vi "Text control 2 v2.9.vi"() -> ()   [LabVIEW 2016]
panel:
  in  "Start Time":dbl caption="Set Start Time (s)"
  out "Total lines":i32
  out "Line running":i32
  in  "byte count":u32=64
  in  "Serial Settings:Serial End Mode for Reads":u16(ring)=2 items=["None", "LastBit", "TermChar"]
  in  "Timeout (ms)":u32=10000
  in  "Enable Termination\nChar (T)":bool=TRUE
  in  "Termination char\n(0xA = '\\n' = LF)\n(0xD = '\\r' = CR)":u8=13 format="%.0x"
  in  "flow control":u16(ring) items=["None"=0, "XON/XOFF"=1, "RTS/CTS"=2, "DTR/DSR"=4]
  in  "stop bits":u16(ring)=10 items=["1.0"=10, "1.5"=15, "2.0"=20]
  in  "parity":u16(ring) items=["None", "Odd", "Even", "Mark", "Space"]
  in  "data bits":u16=8 min=5 max=8 step=1
  in  "VISA resource name":refnum<visa-resource-name>="COM6"
  in  "baud rate":u32=9600
  out "Serial port output":string
  out "error out":errorcluster
  in  "Units":u16(ring) items=["Seconds", "Minutes", "Hours"]
  out "Elapsed Time":dbl caption="Elapsed Time (s)"
  out "Id max vs time":cluster{"Y data in":dbl[], "X data in":dbl[]}[](graph)
  out "Ig":dbl format="%.2e"
  out "Id":dbl format="%.2e"
  out "Is":dbl format="%.2e"
  out "I vs Vg":cluster{"Y data in":dbl[], "X data in":dbl[]}[](graph)
  in  "Panel Controls 2":T1={"Emergency Stop"=refnum, "TransGraph Max"=1e-05, "Text/Graph (text=false)"=TRUE, "TransGraph Min"=1e-11} {"TransGraph Min" format="%.2e"; "TransGraph Max" format="%.2e"}
  out "Command running:":string="#output s 0 0 0 -0.008 0.008 0.002"
  in  "Standby":T2
  in  "Full Reset":bool
  in  "SMU4":cluster{"on/off":bool, "Voltage":dbl} {"Voltage" min=-100.0 max=100.0 format="%.2f"}
  in  "Source/Drain Range":u8(slide)=6 max=11 scale=0.0..11.0
  in  "Source/Drain\nRange mode":u16(ring) items=["Auto", "Limited", "Fixed"]
  in  "Gate Range":u8(slide)=6 max=11 scale=0.0..11.0
  in  "Gate Range\nmode":u16(ring) items=["Auto", "Limited", "Fixed"]
  in  "Gate":T3={"Gate Start"=0.0, "Gate Stop"=2.0, "Gate Step (linear only)"=1.0, "Gate Compliance"=0.0001, "Gate PComp"=0.0, "Range mode"=0, "Range"=6} {"Range" max=11 scale=0.0..11.0; "Range mode" items=["Auto", "Limited", "Fixed"]; "Gate PComp" format="%^.2e"; "Gate Compliance" format="%^.2e"; "Gate Step (linear only)" format="%^.4e"; "Gate Stop" format="%^.4e"; "Gate Start" format="%^.4e"}
  in  "Drain 2":T4={"Drain Start"=0.0, "Drain Stop"=2.0, "Drain Compliance"=0.0001, "Drain Step"=1.0, "Drain PComp"=0.0, "Range mode"=0, "Range"=6} {"Range" max=11 scale=0.0..11.0; "Range mode" items=["Auto", "Limited", "Fixed"]; "Drain PComp" format="%^.2e"; "Drain Step" format="%^.4e"; "Drain Compliance" format="%^.2e"; "Drain Stop" format="%^.4e"; "Drain Start" format="%^.4e"}
  in  "Timings 2":T5={"integration time"=0, "Short/Long integration time"=0.00064, "hold time (sec)"=0.0, "delay time (sec)"=0.0, "Step Time (0 disables)"=0.0, "sweep method"=0, "Pulse period"=0.005, "Base voltage"=0.0, "Pulse width"=0.0005} {"Pulse width" min=0.0005 max=0.1 step=0.0001 format="%.4f"; "Base voltage" format="%^.4e"; "Pulse period" min=0.005 max=1.0 step=0.0001 format="%.4f"; "sweep method" items=["Continuous", "Pulsed"]; "Step Time (0 disables)" format="%.2f"; "delay time (sec)" format="%.4f"; "hold time (sec)" format="%.4f"; "Short/Long integration time" format="%^.0e"; "integration time" scale=0.0..2.0}
  in  "Panel Controls":T6={"Emergency Stop"=refnum, "TransGraph Max"=1e-05, "Text/Graph (text=false)"=TRUE} {"TransGraph Max" format="%.2e"}
  in  "Interrupt run":bool
  in  "Drain: Compliance":dbl=0.001 format="%.8f"
  in  "Gate: Compliance":dbl=0.001 format="%.8f"
  out "Path":path=path "C:/users/rlp38/09Apr2009LTtesting/test2.txt"
  in  "hold time /s":dbl format="%.2f"
  in  "delay time /s":dbl format="%.2f"
  in  "integration time":u32(slide) max=2 step=1 scale=0.0..2.0
  in  "Integration time (short)":dbl=0.0019 min=8e-05 max=0.0019 step=8e-05 format="%^.0e"
  in  "Integration time (long)":dbl=0.32 min=0.04 max=2.0 step=0.02 format="%.2f"
  in  "Step delay /s":dbl format="%.2f"
  in  "Program":string="#pulsedstressV d 0.03 20 0 0.5 0.0827 5\n#\n#itime s\n#gaterangemode l\n#drainrangemode l\n#pulsed on 0.05 0 0.02\n#transfer d 1 -1 -0.1 -1 -1 0\n#wait-min 1\n#transfer d 1 -1 -0.1 -1 -1 0\n#output d 0 -1 -0.5 0 -1 -0.1\n#transfer d -10 40 1 5 40 35\n#transfer d -10 40 1 5 40 35\n#output d 0 40 20 0 40 1\n#\n#\n#sample 1 0.008 221 6 0.003\n#samplei 400e-6 200 6 0.002 0.1\n#vsu2pulse -10 4\n#\n#stressV 0.016 0.03 2e-4 0.1e-3 11\n#stressI 220e-7 0.08 15\n#transfer s -1 1 0.5 -0.005 0.005 0.005\n#output s 0 0 0 -0.008 0.008 0.002\n"
  # "Serial port settings"
  # "Time"
  # "100 samples is approx 13s with medium integration"
  # "Syntax:\nitime [s|m|l]\ngaterangemode [a|l|f]\ndrainrangemode [a|l|f]\npulsed [on|off] PulsePeriod(sec) PulseBaseVoltage PulseONWidth(sec)\nstandby [on l off]\nwait NumMilliseconds\nwait-min NumMinutes\n# texthere = comment\ntransfer [s|d] VgStart VgStop VgStep VdStart VdStop VdStep\noutput [s|d] VgStart VgStop VgStep VdStart VdStop VdStep\nsample Vg Vd NumSamples Time(s) SampleInterval(s)\nsamplei Idg NumSamples Time(s) SampleInterval(s) VDGcompliance\n# if in doubt use SampleInterval(s) = 0.004\nstressV VG VD IGcompliance IDcompliance Duration(sec)\nstressI IDG VDGcompliance Duration(sec)\nvsu2pulse Bias Duration(s)\npulsedstressV [s|d] VEstop VgON VgOFF Period(s) PulseONwidth(s) Vd\nsample-fpp Vg Vd NumSamples Time\nresample-fpp Vg Vd\ntransfer-fpp [s|d] VgStart VgStop VgStep VdStart VdStop VdStep\noutput-fpp [s|d] VgStart VgStop VgStep VdStart VdStop VdStep\nserial SerialPortCommand"
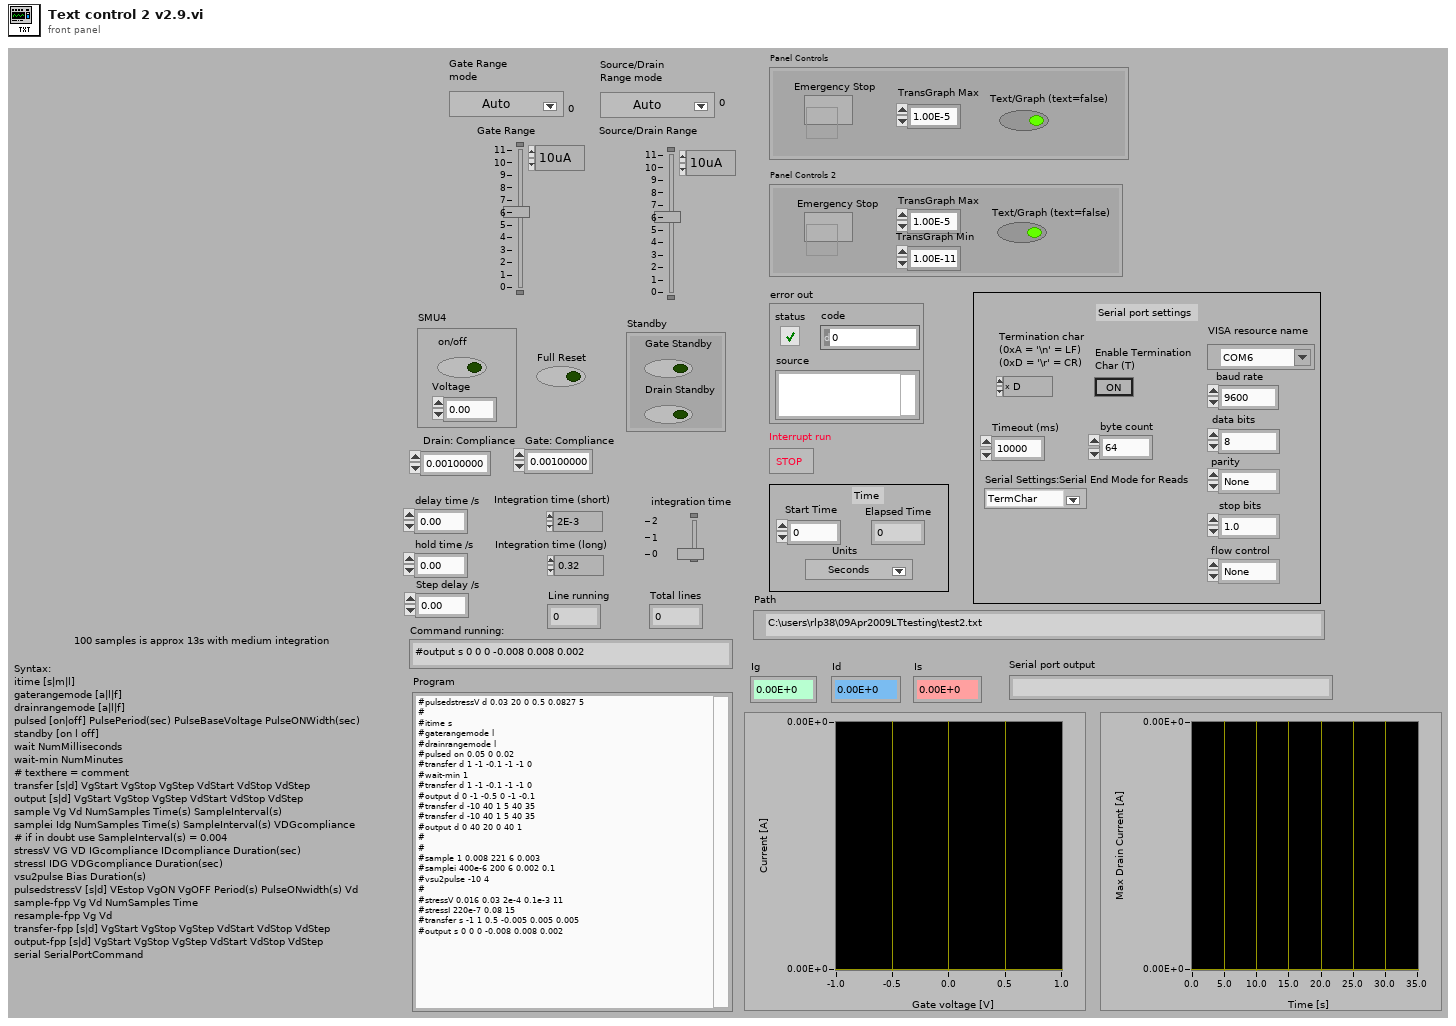
[diagram p1: front panel]
types:
  T1 = cluster{"Emergency Stop":refnum<vi>, "TransGraph Max":dbl, "Text/Graph (text=false)":bool, "TransGraph Min":dbl}
  T2 = cluster{"Gate Standby":bool, "Drain Standby":bool}
  T3 = cluster{"Gate Start":dbl, "Gate Stop":dbl, "Gate Step (linear only)":dbl, "Gate Compliance":dbl, "Gate PComp":dbl, "Range mode":u16, "Range":u8}
  T4 = cluster{"Drain Start":dbl, "Drain Stop":dbl, "Drain Compliance":dbl, "Drain Step":dbl, "Drain PComp":dbl, "Range mode":u16, "Range":u8}
  T5 = cluster{"integration time":u32, "Short/Long integration time":dbl, "hold time (sec)":dbl, "delay time (sec)":dbl, "Step Time (0 disables)":dbl, "sweep method":u16, "Pulse period":dbl, "Base voltage":dbl, "Pulse width":dbl}
  T6 = cluster{"Emergency Stop":refnum<vi>, "TransGraph Max":dbl, "Text/Graph (text=false)":bool}
  T7 = enum16{"open", "replace", "create", "open or create", "replace or create", "replace or create with confirmation"}
  T8 = cluster{"V2 Start":dbl, "V2 Step":dbl, "Number of points":i32}
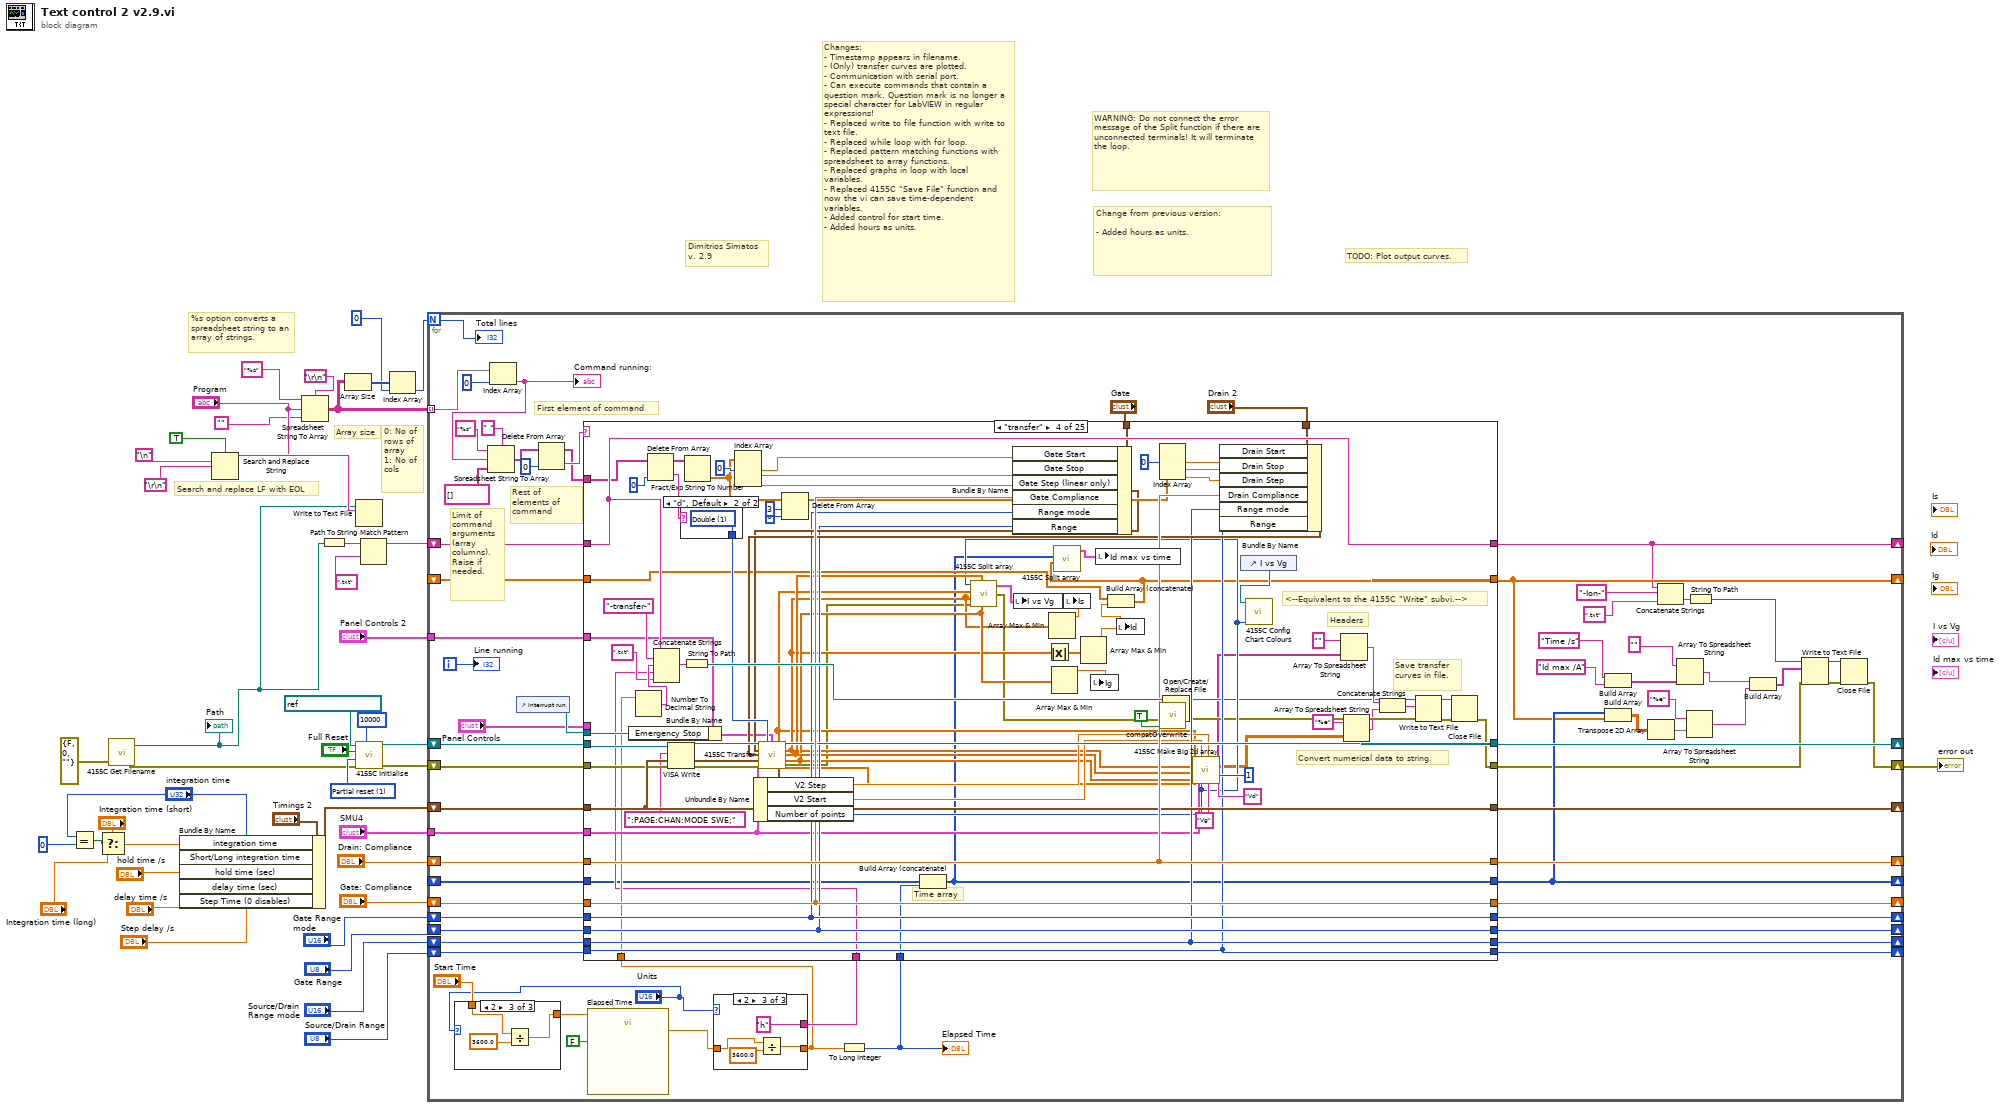
[diagram p0: block diagram]
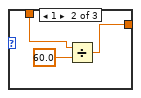
[diagram p3: hidden frame]
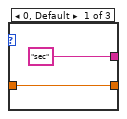
[diagram p4: hidden frame]
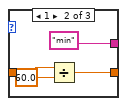
[diagram p5: hidden frame]
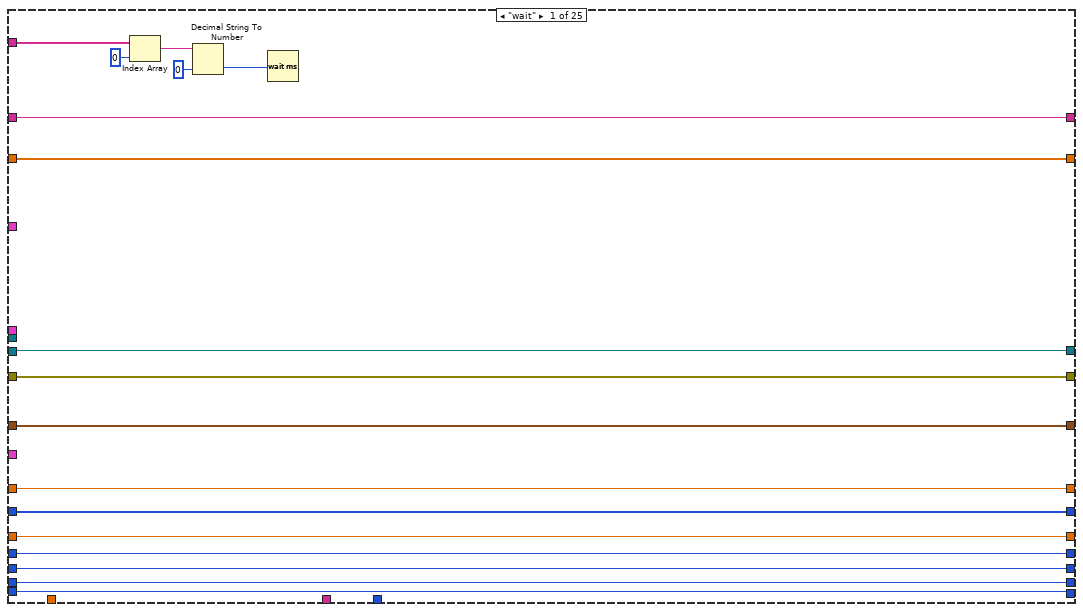
[diagram p6: hidden frame]
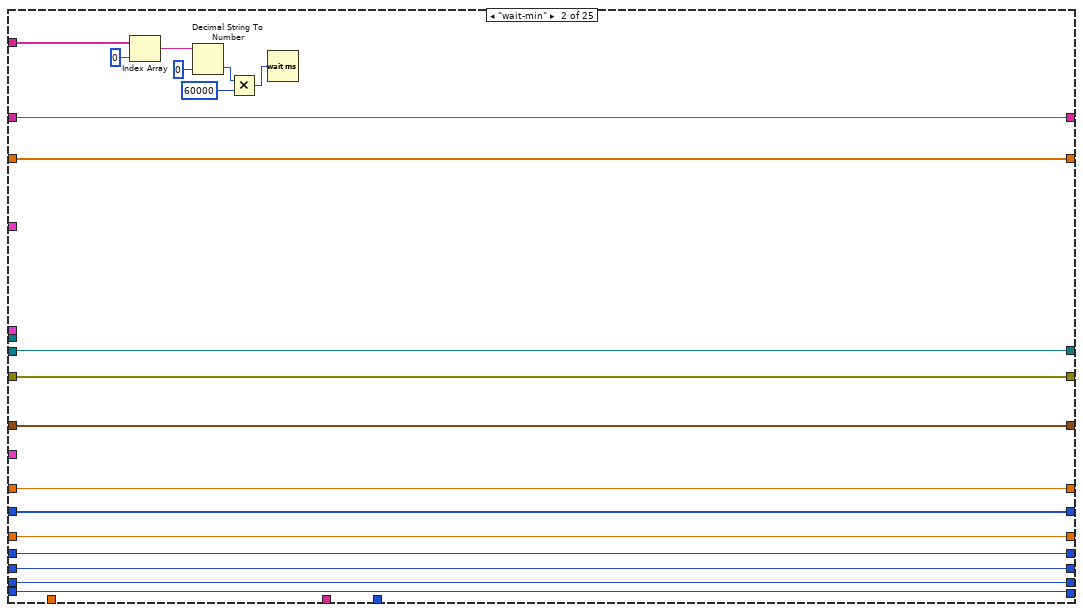
[diagram p7: hidden frame]
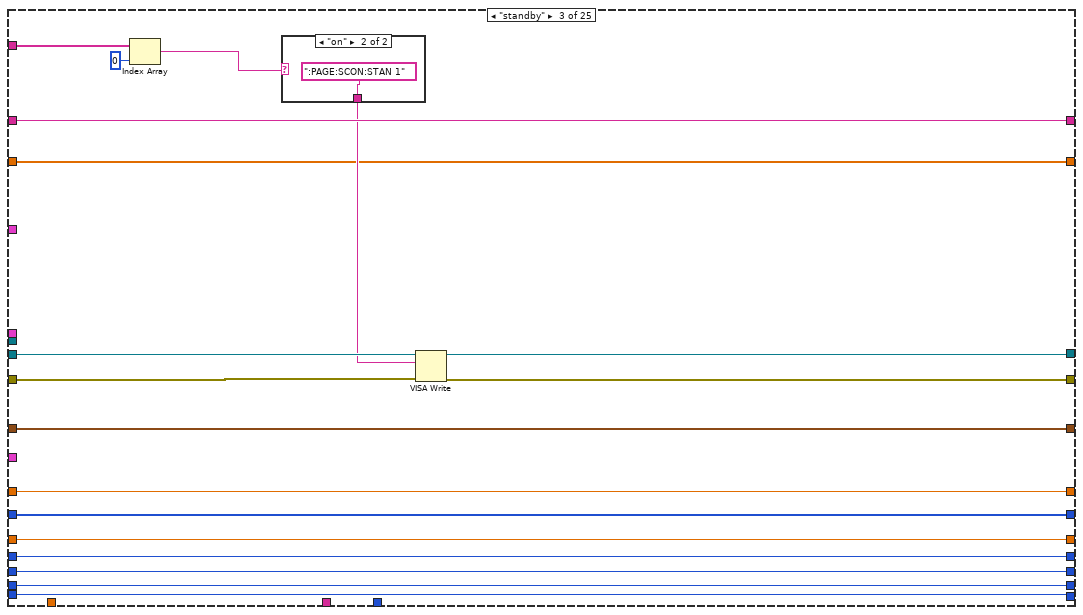
[diagram p8: hidden frame]
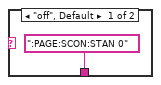
[diagram p9: hidden frame]
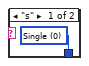
[diagram p10: hidden frame]
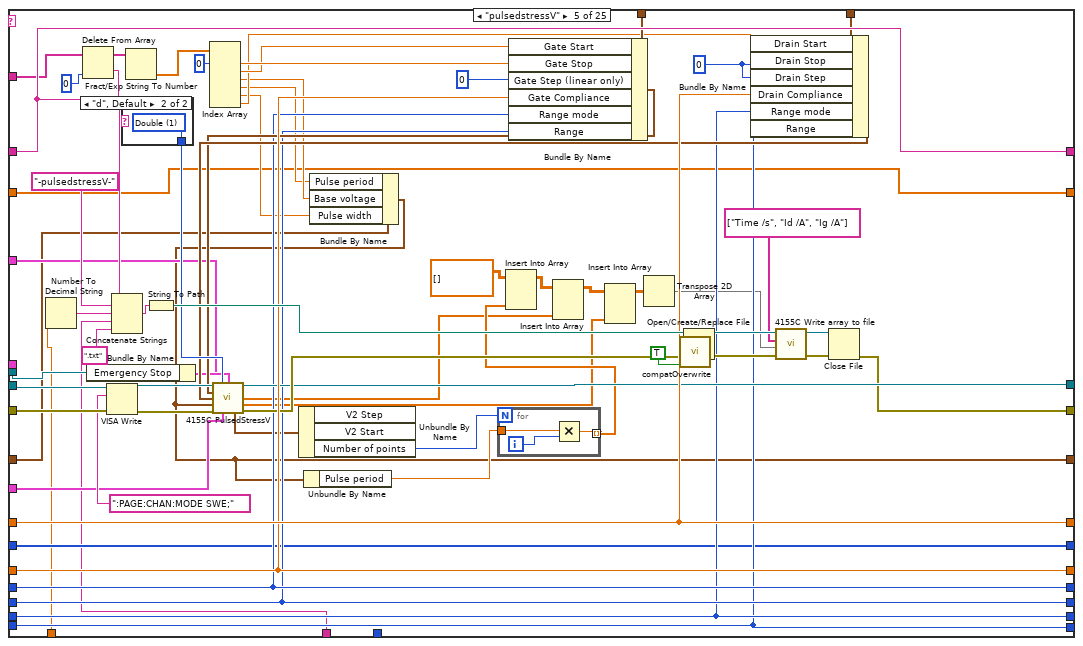
[diagram p11: hidden frame]
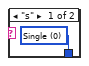
[diagram p12: hidden frame]
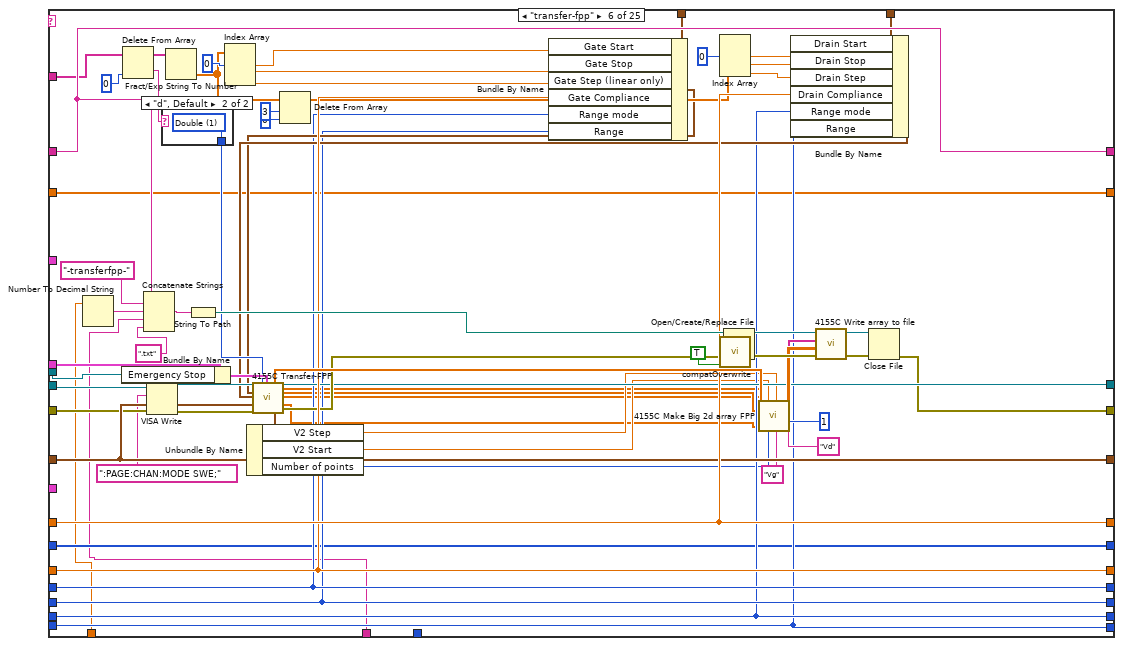
[diagram p13: hidden frame]
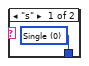
[diagram p14: hidden frame]
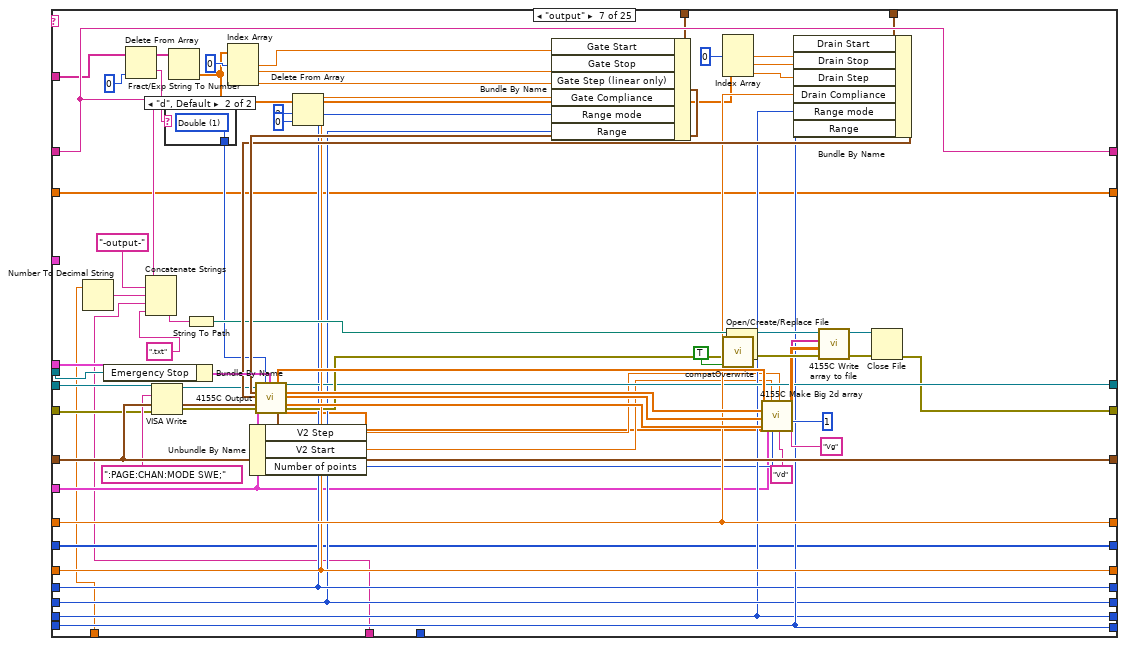
[diagram p15: hidden frame]
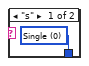
[diagram p16: hidden frame]
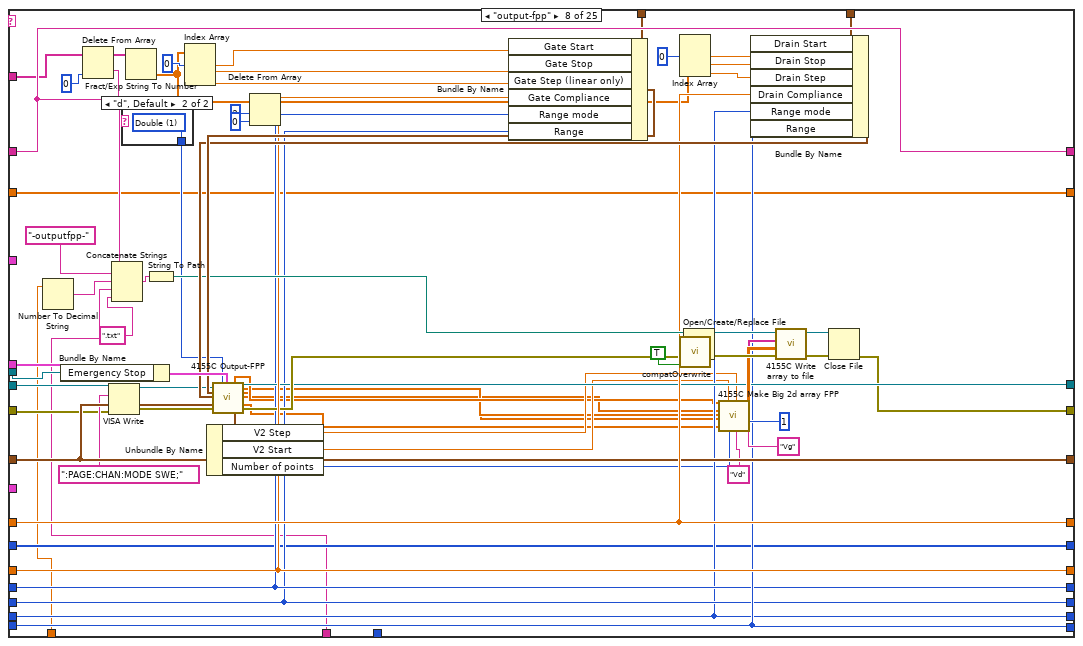
[diagram p17: hidden frame]
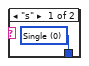
[diagram p18: hidden frame]
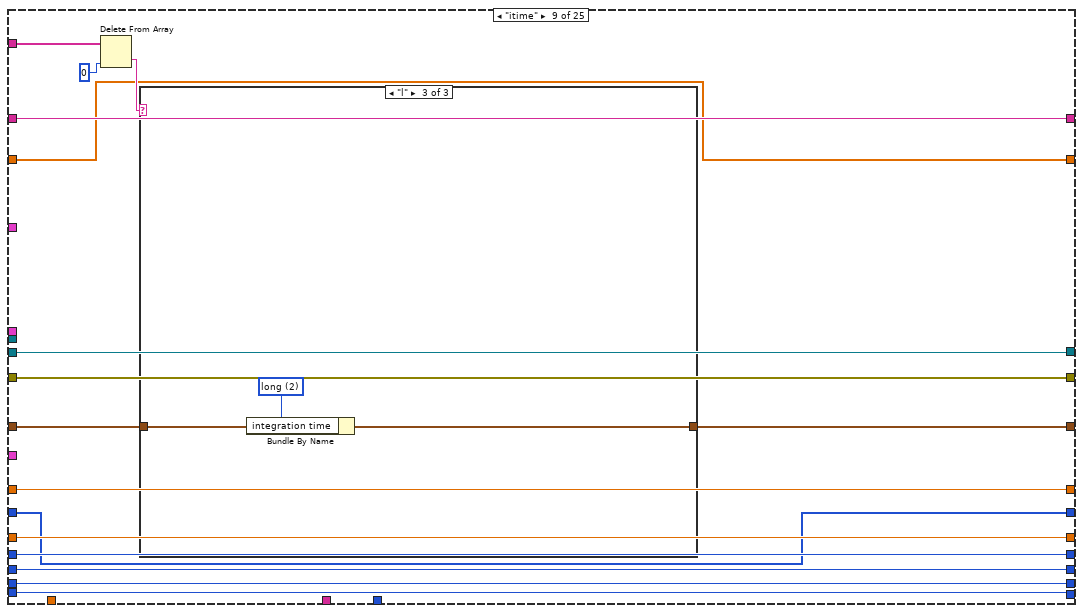
[diagram p19: hidden frame]
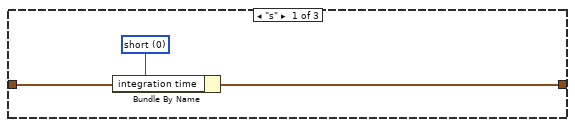
[diagram p20: hidden frame]
diagram:
  w35 = u16 1 items=["Reset All", "Partial reset"] ("Type of reset")
  # "TODO: Plot output curves."
  # "WARNING: Do not connect the error message of the Split function if there are unconnected terminals! It will terminate the loop."
  # "Array size"
  # "%s option converts a spreadsheet string to an array of strings."
  # "0: No of rows of array\n1: No of cols"
  # "Change from previous version:\n\n- Added hours as units."
  # "Dimitrios Simatos\nv. 2.9"
  # "Changes:\n- Timestamp appears in filename.\n- (Only) transfer curves are plotted.\n- Communication with serial port.\n- Can execute commands that contain a question mark. Question mark is no longer a special character for LabVIEW in regular expressions!\n- Replaced write to file function with write to text file.\n- Replaced while loop with for loop.\n- Replaced pattern matching functions with spreadsheet to array functions.\n- Replaced graphs in loop with local variables.\n- Replaced 4155C \"Save File\" function and now the vi can save time-dependent variables.\n- Added control for start time.\n- Added hours as units."
  # "Search and replace LF with EOL"
  n1 = Equal?(x="integration time", y=u32 0) -> (x = y?=w39:bool)
  n2 = Select(t="Integration time (short)", s=w39, f="Integration time (long)") -> (s? t:f=w43:dbl)
  n3 = call "4155C Get Filename.vi"("error in (no error)"=errorcluster {"status"=FALSE, "code"=0, "source"=""}) -> ("error out"=w30:errorcluster, "path"=w2:path)  [unwired: 2 in, 1 out]
  "Path" <- w2
  n4 = Bundle By Name(cluster="Timings 2", "integration time"="integration time", "Short/Long integration time"=w43, "hold time (sec)"="hold time /s", "delay time (sec)"="delay time /s", "Step Time (0 disables)"="Step delay /s") -> (w27:T5)
  n5 = Search and Replace String(replace all?=TRUE ("replace all? (F)"), input string="Program", search string="\n", replace string="\r\n") -> (result string=w17:string)  [unwired: 4 in, 3 out]
  n6 = Spreadsheet String To Array(delimiter (Tab)="\r\n", format string="%s", spreadsheet string="Program", array type (2D Dbl)="") -> (array=w8:string[][])
  n7 = Path To String(path=w2) -> (string=w5:string)
  n8 = Array Size(array=w8) -> (size(s)=w12:i32[])
  n9 = Write to Text File(file (use dialog)=w2, text=w17) -> ()  [unwired: 2 in, 3 out]
  n10 = call "4155C Initialise.vi"("VISA resource name in"=refnum<visa-resource-name> "GPIB0::14::INSTR", "Reset"="Full Reset", "Type of reset"=w35, "error in (no error)"=w30, "VISA Timeout Value"=u32 10000) -> ("VISA Resource Name out"=w29:refnum<visa-resource-name>, "error out"=w28:errorcluster)
  n11 = Match Pattern(string=w5, regular expression=".txt") -> (before substring=w3:string)  [unwired: 1 in, 3 out]
  n12 = Index Array(array=w12, index=0) -> (element=w10:i32)
  n13 = for {
    N: w10 -> [w77]
    tunnel: "SMU4" -> [w89]
    shift-left: "Source/Drain Range" -> [w94]
    shift-right: [w90] -> _
    shift-left: "Source/Drain\nRange mode" -> [w95]
    shift-right: [w91] -> _
    shift-left: "Gate Range" -> [w96]
    shift-right: [w92] -> _
    shift-left: "Gate Range\nmode" -> [w97]
    shift-right: [w93] -> _
    shift-left: "Gate: Compliance" -> [w106]
    shift-right: [w102] -> _
    shift-left: "Drain: Compliance" -> [w107]
    shift-right: [w103] -> _
    shift-left: w27 -> [w108]
    shift-right: [w104] -> _
    shift-left: w28 -> [w109]
    shift-right: [w45] -> w1
    shift-left: w29 -> [w110]
    shift-right: [w105] -> _
    shift-left: w3 -> [w111]
    shift-right: [w50] -> _
    tunnel: "Panel Controls 2" -> [w88]
    shift-right: [w53] -> _
    shift-left: _ -> [w87]
    shift-right: [w54] -> _
    shift-left: _ -> [w83]
    tunnel: w8 -> [w80] mode=indexing
    i -> [w78]
    # "Limit of command arguments (array columns). Raise if needed."
    # "Rest of elements of command"
    # "First element of command"
    n14 = case shown="2" "Units" {
      tunnel: "Start Time" -> [w112 w114 w117]
      tunnel: [w112 w113 w116] -> w48
      frame 0, Default {
      }
      frame 1 {
        n15 = Divide(x=w114, y=60.0) -> (x/y=w113:dbl)
      }
      frame 2 {
        n16 = Divide(x=w117, y=3600.0) -> (x/y=w116:dbl)
      }
    }
    n17 = Index Array(array=w80, index=0 ("line index")) -> (element=w73:string)
    "Command running:" <- w73
    n18 = Spreadsheet String To Array(delimiter (Tab)=" ", format string="%s", spreadsheet string=w73, array type (2D Dbl)=string[] []) -> (array=w70:string[])
    n19 = control-ref of="Interrupt run"() -> (w101:refnum<vi>)
    n20 = Delete From Array(array=w70, index=0) -> (deleted portion=w71:string, array with subset deleted=w69:string[])  [unwired: 1 in]
    n21 = call "Elapsed Time"("Time Target (s)"=w48, "Auto Reset"=FALSE) -> ("Elapsed Time (s)"=w84:dbl)  [unwired: 10 in, 7 out]
    n22 = case shown="2" "Units" {
      tunnel: ["sec" "min" "h"] -> w85
      tunnel: [w119 w123 w126] -> w82
      tunnel: w84 -> [w119 w122 w127]
      frame 0, Default {
      }
      frame 1 {
        n23 = Divide(x=w122, y=60.0) -> (x/y=w123:dbl)
      }
      frame 2 {
        n24 = Divide(x=w127, y=3600.0) -> (x/y=w126:dbl)
      }
    }
    n25 = To Long Integer(number=w82) -> (32bit integer=w81:i32)
    "Elapsed Time" <- w81
    n26 = case shown="\"transfer\"" w71 {
      tunnel: w69 -> [w145 w164 w182 w259 w323 w392 w459 w534 w572 w598 w625 w650 w671 w685 _ _ w789 w850 _ w915 w959 w1001 w1071 w1133 w1140]
      tunnel: w111 -> [w140 w160 w180 w266 w330 w400 w467 w542 w561 w587 w617 w643 w665 w678 w697 w739 w767 w832 w863 w902 w946 w989 w1065 w1129 w1142]
      tunnel: w110 -> [w139 w159 w171 w237 w314 w369 w435 w510 w562 w588 w618 w644 w666 w679 w702 w741 w795 w856 w867 w921 w965 w1007 w1077 w1087 w1146]
      tunnel: w109 -> [w138 w158 w170 w236 w313 w368 w432 w507 w563 w589 w619 w645 w667 w680 w701 w712 w794 w855 w866 w920 w964 w1006 w1076 w1086 w1145]
      tunnel: w108 -> [w137 w157 w179 w262 w289 w396 w463 w538 w571 w597 w616 w642 w664 w677 w700 w736 w758 w824 w872 w895 w939 w982 w1064 w1128 w1147]
      tunnel: w107 -> [w136 w156 w178 w264 w328 w398 w465 w540 w570 w596 w624 w649 w670 w684 w699 w721 w793 w854 w875 w919 w963 w1005 w1075 w1137 w1148]
      tunnel: w106 -> [w135 w155 w177 w263 w327 w397 w464 w539 w569 w595 w623 w648 w669 w683 w698 w722 w768 w833 w874 w903 w947 w990 w1066 w1130 w1150]
      tunnel: [w139 w159 w169 w261 w325 w394 w461 w536 w562 w588 w618 w644 w666 w679 w702 w741 w759 w806 w865 w896 w940 w983 w1017 w1089 w1146] -> w105
      tunnel: [w138 w158 w168 w260 w324 w393 w460 w535 w563 w589 w619 w645 w667 w680 w701 w711 w769 w807 w864 w904 w948 w991 w1016 w1088 w1144] -> w46
      tunnel: [w137 w157 w179 w262 w285 w396 w463 w538 w564 w590 w616 w642 w664 w677 w700 w736 w758 w824 w872 w895 w939 w982 w1064 w1128 w1147] -> w104
      tunnel: [w136 w156 w178 w264 w328 w398 w465 w540 w570 w596 w624 w649 w670 w684 w699 w721 w793 w854 w875 w919 w963 w1005 w1075 w1137 w1148] -> w103
      tunnel: [w135 w155 w177 w263 w327 w397 w464 w539 w569 w595 w623 w648 w669 w683 w698 w722 w768 w833 w874 w903 w947 w990 w1066 w1130 w1150] -> w102
      tunnel: [w140 w160 w180 w266 w330 w400 w467 w542 w561 w587 w617 w643 w665 w678 w697 w739 w767 w832 w863 w902 w946 w989 w1065 w1129 w1142] -> w50
      tunnel: w101 -> [_ _ _ w269 w334 w405 w475 w546 _ _ _ _ _ _ _ _ w764 w829 _ w901 w945 w988 w1037 w1105 _]
      tunnel: "Gate" -> [_ _ _ w246 w317 w379 w446 w521 _ _ _ _ _ _ _ _ _ _ _ _ _ _ _ _ _]
      tunnel: "Drain 2" -> [_ _ _ w245 w316 w378 w445 w520 _ _ _ _ _ _ _ _ _ _ _ _ _ _ _ _ _]
      tunnel: "Panel Controls" -> [_ _ _ _ _ w377 w444 w519 _ _ _ _ _ _ _ _ _ _ _ _ _ _ _ _ _]
      tunnel: w97 -> [w134 w154 w176 w230 w307 w362 w430 w505 w568 w594 _ w641 w663 w676 w696 w723 w754 w820 w868 w891 w935 w978 w1060 w1124 w1151]
      tunnel: w96 -> [w133 w153 w175 w229 w306 w361 w429 w504 w567 w593 w622 _ w654 w682 w695 w724 w755 w821 w869 w892 w936 w979 w1061 w1125 w1152]
      tunnel: w95 -> [w132 w152 w174 w228 w305 w360 w428 w503 w566 w592 w621 w647 w668 _ w694 w725 w756 w822 w870 w893 w937 w980 w1062 w1126 w1153]
      tunnel: w94 -> [w131 w151 w173 w227 w304 w359 w431 w506 w565 w591 w620 w646 _ w681 w693 w726 w757 w823 w871 w894 w938 w981 w1063 w1127 w1154]
      tunnel: [w134 w154 w176 w230 w307 w362 w430 w505 w568 w594 w615 w641 w663 w676 w696 w723 w754 w820 w868 w891 w935 w978 w1060 w1124 w1151] -> w93
      tunnel: [w133 w153 w175 w229 w306 w361 w429 w504 w567 w593 w622 w633 w654 w682 w695 w724 w755 w821 w869 w892 w936 w979 w1061 w1125 w1152] -> w92
      tunnel: [w132 w152 w174 w228 w305 w360 w428 w503 w566 w592 w621 w647 w668 w675 w694 w725 w756 w822 w870 w893 w937 w980 w1062 w1126 w1153] -> w91
      tunnel: [w131 w151 w173 w227 w304 w359 w431 w506 w565 w591 w620 w646 w655 w681 w693 w726 w757 w823 w871 w894 w938 w981 w1063 w1127 w1154] -> w90
      tunnel: w89 -> [_ _ _ w222 w301 _ w423 _ _ _ _ _ _ _ _ _ _ _ _ _ _ _ _ _ _]
      tunnel: w88 -> [_ _ _ w220 w300 _ _ _ _ _ _ _ _ _ _ _ _ _ _ _ _ _ _ _ _]
      tunnel: [w130 w147 w166 w188 w277 w349 w420 w492 w560 w585 w614 w632 w653 w674 w692 w707 w746 w804 w862 w880 w928 w972 w1014 w1082 w1143] -> w53
      tunnel: w87 -> [w130 w147 w166 w211 w277 w349 w420 w492 w560 w585 w614 w632 w653 w674 w692 w707 w746 w804 w862 w880 w928 w972 w1014 w1082 w1143]
      tunnel: w82 -> [_ _ _ w207 w274 w347 w417 w489 _ _ _ _ _ _ _ w705 w744 w801 _ w877 w925 w969 w1011 w1078 _]
      tunnel: w85 -> [_ _ _ w204 w273 w345 w416 w488 _ _ _ _ _ _ _ w703 w742 w800 _ w876 w924 w968 w1010 w1079 _]
      tunnel: w81 -> [_ _ _ w189 _ _ _ _ _ _ _ _ _ _ _ _ _ _ _ _ _ _ _ _ _]
      tunnel: [w129 w146 w165 w187 w276 w348 w419 w491 w559 w584 w613 w631 w652 w673 w691 w706 w745 w803 w861 w879 w927 w971 w1013 w1081 w1149] -> w54
      tunnel: w83 -> [w129 w146 w165 w203 w276 w348 w419 w491 w559 w584 w613 w631 w652 w673 w691 w706 w745 w803 w861 w879 w927 w971 w1013 w1081 w1149]
      frame "wait" {
        n27 = Index Array(array=w145, index=0 ("Index")) -> (element=w143:string)
        n28 = Decimal String To Number(string=w143, default (0L)=u32 0) -> (number=w142:u32)  [unwired: 1 in, 1 out]
        n29 = Wait (ms)(milliseconds to wait=w142) -> ()  [unwired: 1 out]
      }
      frame "wait-min" {
        n30 = Index Array(array=w164, index=0 ("Index")) -> (element=w162:string)
        n31 = Decimal String To Number(string=w162, default (0L)=u32 0) -> (number=w150:u32)  [unwired: 1 in, 1 out]
        n32 = Multiply(x=w150, y=u32 60000) -> (x*y=w149:u32)
        n33 = Wait (ms)(milliseconds to wait=w149) -> ()  [unwired: 1 out]
      }
      frame "standby" {
        n34 = Index Array(array=w182, index=0 ("Index")) -> (element=w172:string)
        n35 = case shown="\"on\"" w172 {
          tunnel: [":PAGE:SCON:STAN 0" ":PAGE:SCON:STAN 1"] -> w167
          frame "off", Default {
          }
          frame "on" {
          }
        }
        n36 = VISA Write(VISA resource name=w171, write buffer=w167, error in (no error)=w170) -> (VISA resource name out=w169:refnum<visa-resource-name>, error out=w168:errorcluster)  [unwired: 1 out]
      }
      frame "transfer" {
        # "<--Equivalent to the 4155C \"Write\" subvi.-->"
        # "Headers"
        # "Convert numerical data to string."
        # "Save transfer curves in file."
        # "Time array"
        n37 = Bundle By Name(cluster=w220, "Emergency Stop"=w269) -> (w221:T1)
        n38 = Number To Decimal String(number=w207) -> (decimal integer string=w206:string)  [unwired: 1 in]
        n39 = Delete From Array(array=w259, index=0 ("Index")) -> (deleted portion=w257:string, array with subset deleted=w256:string[])  [unwired: 1 in]
        n40 = Concatenate Strings(w266, "-transfer-" ("Prefix"), w206, w204, ".txt" ("Suffix")) -> (w268:string)
        n41 = VISA Write(VISA resource name=w237, write buffer=":PAGE:CHAN:MODE SWE;" ("write buffer (\"\")"), error in (no error)=w236) -> (VISA resource name out=w234:refnum<visa-resource-name>, error out=w235:errorcluster)  [unwired: 1 out]
        n42 = case shown="\"d\", Default" w257 {
          tunnel: [w271 w272] -> w255
          frame "s" {
            w271 = u16 0 items=["Single", "Double"] ("sweep mode")
          }
          frame "d", Default {
            w272 = u16 1 items=["Single", "Double"] ("sweep mode")
          }
        }
        n43 = String To Path(string=w268) -> (path=w265:path)
        n44 = Fract/Exp String To Number(string=w256) -> (number=w241:dbl[])  [unwired: 3 in, 1 out]
        n45 = Index Array(array=w241, index #1=0 ("Index")) -> (element #1=w254:dbl, element #2=w253:dbl, element #3=w252:dbl)  [unwired: 2 in]
        n46 = Delete From Array(array=w241, length=3 ("Length"), index=0 ("Index")) -> (array with subset deleted=w239:dbl[])  [unwired: 1 out]
        n47 = Build Array (concatenate)(w203, w189) -> (w187:i32[])
        n48 = Bundle By Name(cluster=w246, "Gate Start"=w254, "Gate Stop"=w253, "Gate Step (linear only)"=w252, "Gate Compliance"=w263, "Range mode"=w230, "Range"=w229) -> (w231:T3)
        n49 = Index Array(array=w239, index #1=0 ("Index")) -> (element #1=w249:dbl, element #2=w248:dbl, element #3=w247:dbl)  [unwired: 2 in]
        n50 = call <vilib>:"compatOverwrite.vi"("overwrite (F)"=TRUE) -> ("overwrite?"=w219:T7)
        n51 = Bundle By Name(cluster=w245, "Drain Start"=w249, "Drain Stop"=w248, "Drain Step"=w247, "Drain Compliance"=w264, "Range mode"=w228, "Range"=w227) -> (w232:T4)
        n52 = call "4155C Transfer.vi"("VISA resource name in"=w234, "Gate"=w231, "Drain"=w232, "Timings"=w262, "error in (no error)"=w235, "SMU4"=w222, "sweep mode"=w255, "Panel Controls"=w221) -> ("VG"=w212:dbl[], "Outparams"=w226:T8, "VISA Resource Name out"=w261:refnum<visa-resource-name>, "IS"=w213:dbl[], "ID"=w218:dbl[], "IG"=w214:dbl[], "error out"=w199:errorcluster, "SMU4"=w223:dbl[])  [unwired: 12 in]
        n53 = Unbundle By Name(w226) -> ("V2 Step"=w225:dbl, "V2 Start"=w224:dbl, "Number of points"=w209:i32)
        n54 = call "4155C Split array.vi"("Number of VAR2 steps"=w209, "Y2 data in"=w218, "X data in"=w212, "Y1 data in"=w213, "Y3 data in"=w214, "error in (no error)"=w199) -> ("Array of clusters"=w202:cluster{"Y data in":dbl[], "X data in":dbl[]}[], "error out"=w200:errorcluster)  [unwired: 1 in]
        n55 = local write "I vs Vg"(w202) -> ()
        n56 = Absolute Value(x=w213) -> (abs(x)=w217:dbl[])
        n57 = Array Max & Min(array=w213) -> (max value=w215:dbl)  [unwired: 3 out]
        n58 = Array Max & Min(array=w214) -> (max value=w216:dbl)  [unwired: 3 out]
        n59 = local write "Is"(w215) -> ()
        n60 = Array Max & Min(array=w217) -> (max value=w210:dbl)  [unwired: 3 out]
        n61 = local write "Ig"(w216) -> ()
        n62 = Build Array (concatenate)(w211, w210) -> (w188:dbl[])
        n63 = call "4155C Split array.vi"("X data in"=w187, "Y1 data in"=w188) -> ("Array of clusters"=w201:cluster{"Y data in":dbl[], "X data in":dbl[]}[])  [unwired: 5 in, 1 out]
        n64 = local write "Id max vs time"(w201) -> ()
        n65 = local write "Id"(w210) -> ()
        n66 = Open/Create/Replace File(file path (use dialog)=w265, error in=w200, operation (0:open)=w219) -> (refnum out=w186:refnum<file>, error out=w196:errorcluster)  [unwired: 3 in, 1 out]
        n67 = call "4155C Make Big 2d array.vi"("1D Var1"=w212, "1d IS"=w213, "1d ID"=w218, "1d IG"=w214, "1d SMU4"=w223, "SMU4"=w222, "VAR2 START"=w224, "Number of VAR2 steps"=w209, "VAR2 STEP"=w225, "VAR1 Name"="Vg", "Decimal places in header"=i8 1, "VAR2 Name"="Vd") -> ("Header array"=w185:string[], "Data array"=w193:dbl[][])  [unwired: 14 in]
        n68 = control-ref of="I vs Vg"() -> (w208:refnum<vi>)
        n69 = call "4155C Config Chart Colours.vi"("Numeric"=w209, "XY Graph 2"=w208) -> ()  [unwired: 6 in]
        n70 = Array To Spreadsheet String(array=w185, 3:"" ("format string")) -> (spreadsheet string=w192:string)  [unwired: 1 in]
        n71 = Array To Spreadsheet String(array=w193, 3:"%e" ("format string")) -> (spreadsheet string=w195:string)  [unwired: 1 in]
        n72 = Concatenate Strings(w192, w195) -> (w194:string)
        n73 = Write to Text File(file (use dialog)=w186, text=w194, error in=w196) -> (refnum out=w198:refnum<file>, error out=w197:errorcluster)  [unwired: 1 in, 1 out]
        n74 = Close File(refnum=w198, error in=w197) -> (error out=w260:errorcluster)  [unwired: 1 out]
      }
      frame "pulsedstressV" {
        w283 = 0
        n75 = Number To Decimal String(number=w274) -> (decimal integer string=w331:string)  [unwired: 1 in]
        n76 = Delete From Array(array=w323, index=0 ("Index")) -> (deleted portion=w321:string, array with subset deleted=w320:string[])  [unwired: 1 in]
        n77 = Bundle By Name(cluster=w300, "Emergency Stop"=w334) -> (w302:T1)
        n78 = VISA Write(VISA resource name=w314, write buffer=":PAGE:CHAN:MODE SWE;" ("write buffer (\"\")"), error in (no error)=w313) -> (VISA resource name out=w311:refnum<visa-resource-name>, error out=w312:errorcluster)  [unwired: 1 out]
        n79 = Concatenate Strings(w330, "-pulsedstressV-" ("Substring"), w331, w273, ".txt" ("Substring")) -> (w333:string)
        n80 = case shown="\"d\", Default" w321 {
          tunnel: [w343 w344] -> w319
          frame "s" {
            w343 = u16 0 items=["Single", "Double"] ("sweep mode")
          }
          frame "d", Default {
            w344 = u16 1 items=["Single", "Double"] ("sweep mode")
          }
        }
        n81 = Fract/Exp String To Number(string=w320) -> (number=w315:dbl[])  [unwired: 3 in, 1 out]
        n82 = String To Path(string=w333) -> (path=w329:path)
        n83 = Index Array(array=w315, index #1=0 ("Index")) -> (element #1=w292:dbl, element #2=w291:dbl, element #3=w288:dbl, element #4=w287:dbl, element #5=w286:dbl, element #6=w290:dbl)  [unwired: 5 in]
        n84 = Bundle By Name(cluster=w289, "Pulse period"=w287, "Base voltage"=w288, "Pulse width"=w286) -> (w285:T5)
        n85 = Unbundle By Name(w285) -> ("Pulse period"=w293:dbl)
        n86 = Bundle By Name(cluster=w317, "Gate Start"=w291, "Gate Stop"=w292, "Gate Step (linear only)"=0, "Gate Compliance"=w327, "Range mode"=w307, "Range"=w306) -> (w308:T3)
        n87 = call <vilib>:"compatOverwrite.vi"("overwrite (F)"=TRUE) -> ("overwrite?"=w278:T7)
        n88 = Bundle By Name(cluster=w316, "Drain Start"=w290, "Drain Stop"=w283, "Drain Step"=w283, "Drain Compliance"=w328, "Range mode"=w305, "Range"=w304) -> (w309:T4)
        n89 = call "4155C PulsedStressV.vi"("VISA resource name in"=w311, "sweep mode"=w319, "Panel Controls"=w302, "Gate"=w308, "Drain"=w309, "Timings"=w285, "error in (no error)"=w312, "SMU4"=w301) -> ("VISA Resource Name out"=w325:refnum<visa-resource-name>, "ID"=w281:dbl[], "IG"=w279:dbl[], "Outparams"=w303:T8, "error out"=w326:errorcluster)  [unwired: 3 in]
        n90 = Unbundle By Name(w303) -> ("Number of points"=w280:i32)  [unwired: 2 out]
        n91 = for {
          N: w280 -> [_]
          tunnel: [w340] -> w282 mode=indexing
          tunnel: w293 -> [w342]
          i -> [w341]
          n92 = Multiply(x=w342, y=w341) -> (x*y=w340:dbl)
        }
        n93 = Insert Into Array(array=dbl[][] [] ("Input Array"), new element=w282) -> (w294:dbl[][])  [unwired: 2 in]
        n94 = Insert Into Array(array=w294, new element=w281) -> (w299:dbl[][])  [unwired: 2 in]
        n95 = Insert Into Array(array=w299, new element=w279) -> (w298:dbl[][])  [unwired: 2 in]
        n96 = Transpose 2D Array(2D array=w298) -> (transposed array=w297:dbl[][])
        n97 = Open/Create/Replace File(file path (use dialog)=w329, error in=w326, operation (0:open)=w278) -> (refnum out=w337:refnum<file>, error out=w338:errorcluster)  [unwired: 3 in, 1 out]
        n98 = call "4155C Write array to file.vi"("Byte Stream File Refnum"=w337, "Header"=string[] ["Time /s", "Id /A", "Ig /A"], "Data Array"=w297, "error in (no error)"=w338) -> ("dup refnum"=w335:refnum<file>, "error out"=w336:errorcluster)  [unwired: 1 in]
        n99 = Close File(refnum=w335, error in=w336) -> (error out=w324:errorcluster)  [unwired: 1 out]
      }
      frame "transfer-fpp" {
        n100 = Number To Decimal String(number=w347) -> (decimal integer string=w401:string)  [unwired: 1 in]
        n101 = Bundle By Name(cluster=w377, "Emergency Stop"=w405) -> (w413:T6)
        n102 = Delete From Array(array=w392, index=0 ("Index")) -> (deleted portion=w390:string, array with subset deleted=w389:string[])  [unwired: 1 in]
        n103 = Concatenate Strings(w400, "-transferfpp-" ("Substring"), w401, w345, ".txt" ("Substring")) -> (w403:string)
        n104 = VISA Write(VISA resource name=w369, write buffer=":PAGE:CHAN:MODE SWE;" ("write buffer (\"\")"), error in (no error)=w368) -> (VISA resource name out=w366:refnum<visa-resource-name>, error out=w367:errorcluster)  [unwired: 1 out]
        n105 = case shown="\"d\", Default" w390 {
          tunnel: [w414 w415] -> w388
          frame "s" {
            w414 = u16 0 items=["Single", "Double"] ("sweep mode")
          }
          frame "d", Default {
            w415 = u16 1 items=["Single", "Double"] ("sweep mode")
          }
        }
        n106 = Fract/Exp String To Number(string=w389) -> (number=w373:dbl[])  [unwired: 3 in, 1 out]
        n107 = String To Path(string=w403) -> (path=w399:path)
        n108 = Index Array(array=w373, index #1=0 ("Index")) -> (element #1=w387:dbl, element #2=w386:dbl, element #3=w385:dbl)  [unwired: 2 in]
        n109 = Delete From Array(array=w373, length=3 ("Length"), index=0 ("Index")) -> (array with subset deleted=w371:dbl[])  [unwired: 1 out]
        n110 = Bundle By Name(cluster=w379, "Gate Start"=w387, "Gate Stop"=w386, "Gate Step (linear only)"=w385, "Gate Compliance"=w397, "Range mode"=w362, "Range"=w361) -> (w363:T3)
        n111 = Index Array(array=w371, index #1=0 ("Index")) -> (element #1=w382:dbl, element #2=w381:dbl, element #3=w380:dbl)  [unwired: 2 in]
        n112 = call <vilib>:"compatOverwrite.vi"("overwrite (F)"=TRUE) -> ("overwrite?"=w350:T7)
        n113 = Bundle By Name(cluster=w378, "Drain Start"=w382, "Drain Stop"=w381, "Drain Step"=w380, "Drain Compliance"=w398, "Range mode"=w360, "Range"=w359) -> (w364:T4)
        n114 = call "4155C Transfer-FPP.vi"("VISA resource name in"=w366, "Gate"=w363, "Drain"=w364, "Timings"=w396, "error in (no error)"=w367, "sweep mode"=w388, "Panel Controls"=w413) -> ("VG"=w404:dbl[], "Outparams"=w358:T8, "VISA Resource Name out"=w394:refnum<visa-resource-name>, "Vprobe2"=w354:dbl[], "ID"=w353:dbl[], "IG"=w352:dbl[], "Vprobe1"=w351:dbl[], "error out"=w395:errorcluster)  [unwired: 13 in]
        n115 = Unbundle By Name(w358) -> ("V2 Step"=w357:dbl, "V2 Start"=w356:dbl, "Number of points"=w355:i32)
        n116 = Open/Create/Replace File(file path (use dialog)=w399, error in=w395, operation (0:open)=w350) -> (refnum out=w410:refnum<file>, error out=w411:errorcluster)  [unwired: 3 in, 1 out]
        n117 = call "4155C Make Big 2d array FPP.vi"("1D Var1"=w404, "1d ID"=w353, "1d Vp2"=w354, "1d IG"=w352, "1d Vp1"=w351, "VAR2 START"=w356, "Number of VAR2 steps"=w355, "VAR2 STEP"=w357, "VAR1 Name"="Vg", "Decimal places in header"=i8 1, "VAR2 Name"="Vd") -> ("Header array"=w406:string[], "Data array"=w407:dbl[][])  [unwired: 15 in]
        n118 = call "4155C Write array to file.vi"("Byte Stream File Refnum"=w410, "Header"=w406, "Data Array"=w407, "error in (no error)"=w411) -> ("dup refnum"=w408:refnum<file>, "error out"=w409:errorcluster)  [unwired: 1 in]
        n119 = Close File(refnum=w408, error in=w409) -> (error out=w393:errorcluster)  [unwired: 1 out]
      }
      frame "output" {
        n120 = Number To Decimal String(number=w417) -> (decimal integer string=w468:string)  [unwired: 1 in]
        n121 = Bundle By Name(cluster=w444, "Emergency Stop"=w475) -> (w485:T6)
        n122 = Delete From Array(array=w459, index=0 ("Index")) -> (deleted portion=w457:string, array with subset deleted=w456:string[])  [unwired: 1 in]
        n123 = Concatenate Strings(w467, "-output-" ("Substring"), w468, w416, ".txt" ("Substring")) -> (w470:string)
        n124 = VISA Write(VISA resource name=w435, write buffer=":PAGE:CHAN:MODE SWE;" ("write buffer (\"\")"), error in (no error)=w432) -> (VISA resource name out=w434:refnum<visa-resource-name>, error out=w433:errorcluster)  [unwired: 1 out]
        n125 = case shown="\"d\", Default" w457 {
          tunnel: [w486 w487] -> w455
          frame "s" {
            w486 = u16 0 items=["Single", "Double"] ("sweep mode")
          }
          frame "d", Default {
            w487 = u16 1 items=["Single", "Double"] ("sweep mode")
          }
        }
        n126 = Fract/Exp String To Number(string=w456) -> (number=w438:dbl[])  [unwired: 3 in, 1 out]
        n127 = String To Path(string=w470) -> (path=w466:path)
        n128 = Index Array(array=w438, index #1=0 ("Index")) -> (element #1=w454:dbl, element #2=w453:dbl, element #3=w452:dbl)  [unwired: 2 in]
        n129 = Delete From Array(array=w438, length=3 ("Length"), index=0 ("Index")) -> (array with subset deleted=w437:dbl[])  [unwired: 1 out]
        n130 = Bundle By Name(cluster=w446, "Gate Start"=w454, "Gate Stop"=w453, "Gate Step (linear only)"=w452, "Gate Compliance"=w464, "Range mode"=w430, "Range"=w429) -> (w484:T3)
        n131 = Index Array(array=w437, index #1=0 ("Index")) -> (element #1=w449:dbl, element #2=w448:dbl, element #3=w447:dbl)  [unwired: 2 in]
        n132 = call <vilib>:"compatOverwrite.vi"("overwrite (F)"=TRUE) -> ("overwrite?"=w421:T7)
        n133 = Bundle By Name(cluster=w445, "Drain Start"=w449, "Drain Stop"=w448, "Drain Step"=w447, "Drain Compliance"=w465, "Range mode"=w428, "Range"=w431) -> (w483:T4)
        n134 = call "4155C Output.vi"("VISA resource name in"=w434, "Gate"=w484, "Drain"=w483, "Timings"=w463, "error in (no error)"=w433, "SMU4"=w423, "sweep mode"=w455, "Panel controls"=w485) -> ("VD"=w471:dbl[], "Outparams"=w426:T8, "VISA Resource Name out"=w461:refnum<visa-resource-name>, "IS"=w474:dbl[], "ID"=w473:dbl[], "IG"=w472:dbl[], "error out"=w462:errorcluster, "SMU4"=w422:dbl[])  [unwired: 12 in]
        n135 = Unbundle By Name(w426) -> ("V2 Step"=w427:dbl, "V2 Start"=w425:dbl, "Number of points"=w424:i32)
        n136 = Open/Create/Replace File(file path (use dialog)=w466, error in=w462, operation (0:open)=w421) -> (refnum out=w480:refnum<file>, error out=w481:errorcluster)  [unwired: 3 in, 1 out]
        n137 = call "4155C Make Big 2d array.vi"("1D Var1"=w471, "1d IS"=w474, "1d ID"=w473, "1d IG"=w472, "1d SMU4"=w422, "SMU4"=w423, "VAR2 START"=w425, "Number of VAR2 steps"=w424, "VAR2 STEP"=w427, "VAR1 Name"="Vd", "Decimal places in header"=i8 1, "VAR2 Name"="Vg") -> ("Header array"=w476:string[], "Data array"=w477:dbl[][])  [unwired: 14 in]
        n138 = call "4155C Write array to file.vi"("Byte Stream File Refnum"=w480, "Header"=w476, "Data Array"=w477, "error in (no error)"=w481) -> ("dup refnum"=w478:refnum<file>, "error out"=w479:errorcluster)  [unwired: 1 in]
        n139 = Close File(refnum=w478, error in=w479) -> (error out=w460:errorcluster)  [unwired: 1 out]
      }
      frame "output-fpp" {
        n140 = Number To Decimal String(number=w489) -> (decimal integer string=w543:string)  [unwired: 1 in]
        n141 = Bundle By Name(cluster=w519, "Emergency Stop"=w546) -> (w556:T6)
        n142 = Delete From Array(array=w534, index=0 ("Index")) -> (deleted portion=w532:string, array with subset deleted=w531:string[])  [unwired: 1 in]
        n143 = VISA Write(VISA resource name=w510, write buffer=":PAGE:CHAN:MODE SWE;" ("write buffer (\"\")"), error in (no error)=w507) -> (VISA resource name out=w509:refnum<visa-resource-name>, error out=w508:errorcluster)  [unwired: 1 out]
        n144 = Concatenate Strings(w542, "-outputfpp-" ("Substring"), w543, w488, ".txt" ("Substring")) -> (w545:string)
        n145 = case shown="\"d\", Default" w532 {
          tunnel: [w557 w558] -> w530
          frame "s" {
            w557 = u16 0 items=["Single", "Double"] ("sweep mode")
          }
          frame "d", Default {
            w558 = u16 1 items=["Single", "Double"] ("sweep mode")
          }
        }
        n146 = Fract/Exp String To Number(string=w531) -> (number=w513:dbl[])  [unwired: 3 in, 1 out]
        n147 = String To Path(string=w545) -> (path=w541:path)
        n148 = Index Array(array=w513, index #1=0 ("Index")) -> (element #1=w529:dbl, element #2=w528:dbl, element #3=w527:dbl)  [unwired: 2 in]
        n149 = Delete From Array(array=w513, length=3 ("Length"), index=0 ("Index")) -> (array with subset deleted=w512:dbl[])  [unwired: 1 out]
        n150 = Bundle By Name(cluster=w521, "Gate Start"=w529, "Gate Stop"=w528, "Gate Step (linear only)"=w527, "Gate Compliance"=w539, "Range mode"=w505, "Range"=w504) -> (w555:T3)
        n151 = Index Array(array=w512, index #1=0 ("Index")) -> (element #1=w524:dbl, element #2=w523:dbl, element #3=w522:dbl)  [unwired: 2 in]
        n152 = call <vilib>:"compatOverwrite.vi"("overwrite (F)"=TRUE) -> ("overwrite?"=w493:T7)
        n153 = Bundle By Name(cluster=w520, "Drain Start"=w524, "Drain Stop"=w523, "Drain Step"=w522, "Drain Compliance"=w540, "Range mode"=w503, "Range"=w506) -> (w554:T4)
        n154 = call "4155C Output-FPP.vi"("VISA resource name in"=w509, "Gate"=w555, "Drain"=w554, "Timings"=w538, "error in (no error)"=w508, "sweep mode"=w530, "Panel controls"=w556) -> ("VD"=w498:dbl[], "Outparams"=w501:T8, "VISA Resource Name out"=w536:refnum<visa-resource-name>, "Vprobe2"=w497:dbl[], "ID"=w496:dbl[], "IG"=w495:dbl[], "Vprobe1"=w494:dbl[], "error out"=w537:errorcluster)  [unwired: 13 in]
        n155 = Unbundle By Name(w501) -> ("V2 Step"=w502:dbl, "V2 Start"=w500:dbl, "Number of points"=w499:i32)
        n156 = Open/Create/Replace File(file path (use dialog)=w541, error in=w537, operation (0:open)=w493) -> (refnum out=w551:refnum<file>, error out=w552:errorcluster)  [unwired: 3 in, 1 out]
        n157 = call "4155C Make Big 2d array FPP.vi"("1D Var1"=w498, "1d ID"=w496, "1d Vp2"=w497, "1d IG"=w495, "1d Vp1"=w494, "VAR2 START"=w500, "Number of VAR2 steps"=w499, "VAR2 STEP"=w502, "VAR1 Name"="Vd", "Decimal places in header"=i8 1, "VAR2 Name"="Vg") -> ("Header array"=w547:string[], "Data array"=w548:dbl[][])  [unwired: 15 in]
        n158 = call "4155C Write array to file.vi"("Byte Stream File Refnum"=w551, "Header"=w547, "Data Array"=w548, "error in (no error)"=w552) -> ("dup refnum"=w549:refnum<file>, "error out"=w550:errorcluster)  [unwired: 1 in]
        n159 = Close File(refnum=w549, error in=w550) -> (error out=w535:errorcluster)  [unwired: 1 out]
      }
      frame "itime" {
        n160 = Delete From Array(array=w572, index=0 ("Index")) -> (deleted portion=w573:string)  [unwired: 1 in, 1 out]
        n161 = case shown="\"l\"" w573 {
          tunnel: w571 -> [w577 w579 w582]
          tunnel: [w576 w578 w581] -> w564
          frame "s" {
            w575 = u32 0 items=["short  ", "medium  ", "long  "] ("integration time 2")
            n162 = Bundle By Name(cluster=w577, "integration time"=w575) -> (w576:T5)
          }
          frame "m", Default {
            w580 = u32 1 items=["short  ", "medium  ", "long  "] ("integration time 2")
            n163 = Bundle By Name(cluster=w579, "integration time"=w580) -> (w578:T5)
          }
          frame "l" {
            w583 = u32 2 items=["short  ", "medium  ", "long  "] ("integration time 2")
            n164 = Bundle By Name(cluster=w582, "integration time"=w583) -> (w581:T5)
          }
        }
      }
      frame "pulsed" {
        n165 = Delete From Array(array=w598, index=0 ("Index")) -> (deleted portion=w599:string, array with subset deleted=w586:string[])  [unwired: 1 in]
        n166 = case shown="\"on\", Default" w599 {
          tunnel: w597 -> [w609 w612]
          tunnel: [w608 w611] -> w590
          tunnel: w586 -> [w606 _]
          frame "on", Default {
            w607 = u16 1 items=["Continuous", "Pulsed"] ("sweep method")
            n167 = Fract/Exp String To Number(string=w606) -> (number=w604:dbl[])  [unwired: 3 in, 1 out]
            n168 = Index Array(array=w604, index #1=0 ("Index")) -> (element #1=w603:dbl, element #2=w602:dbl, element #3=w601:dbl)  [unwired: 2 in]
            n169 = Bundle By Name(cluster=w609, "sweep method"=w607, "Pulse period"=w603, "Base voltage"=w602, "Pulse width"=w601) -> (w608:T5)
          }
          frame "off" {
            w610 = u16 0 items=["Continuous", "Pulsed"] ("sweep method")
            n170 = Bundle By Name(cluster=w612, "sweep method"=w610) -> (w611:T5)
          }
        }
      }
      frame "gaterangemode" {
        n171 = Delete From Array(array=w625, index=0 ("Index")) -> (deleted portion=w626:string)  [unwired: 1 in, 1 out]
        n172 = case shown="\"f\"" w626 {
          tunnel: [w628 w629 w630] -> w615
          frame "a", Default {
            w628 = u16 0 items=["Auto", "Limited", "Fixed"] ("Gate Range\nmode 2")
          }
          frame "f" {
            w629 = u16 2 items=["Auto", "Limited", "Fixed"] ("Gate Range\nmode 2")
          }
          frame "l" {
            w630 = u16 1 items=["Auto", "Limited", "Fixed"] ("Gate Range\nmode 2")
          }
        }
      }
      frame "gaterange" {
        (unwired) u8 11 items=["10fA  ", "100fA  ", "1nA  ", "10nA", "100nA", "1uA", "10uA", "100uA", "1mA", "10mA", "100mA", "1A"] ("Gate Range 2")
        n173 = Delete From Array(array=w650, index=0 ("Index")) -> (deleted portion=w640:string)  [unwired: 1 in, 1 out]
        n174 = Scan Value(string=w640, format string="") -> (value=w638:dbl)  [unwired: 1 in, 1 out]
        n175 = Logarithm Base 10(1:w638) -> (0:w637:dbl)
        n176 = Round To Nearest(number=w637) -> (nearest integer value=w636:dbl)
        n177 = Add(x=w636, y=11.0) -> (x+y=w634:dbl)
        n178 = To Unsigned Byte Integer(number=w634) -> (unsigned 8bit integer=w633:u8)
      }
      frame "drainrange" {
        (unwired) u8 11 items=["10fA  ", "100fA  ", "1nA  ", "10nA", "100nA", "1uA", "10uA", "100uA", "1mA", "10mA", "100mA", "1A"] ("Gate Range 2")
        n179 = Delete From Array(array=w671, index=0 ("Index")) -> (deleted portion=w662:string)  [unwired: 1 in, 1 out]
        n180 = Scan Value(string=w662, format string="") -> (value=w660:dbl)  [unwired: 1 in, 1 out]
        n181 = Logarithm Base 10(1:w660) -> (0:w659:dbl)
        n182 = Round To Nearest(number=w659) -> (nearest integer value=w658:dbl)
        n183 = Add(x=w658, y=11.0) -> (x+y=w656:dbl)
        n184 = To Unsigned Byte Integer(number=w656) -> (unsigned 8bit integer=w655:u8)
      }
      frame "drainrangemode" {
        n185 = Delete From Array(array=w685, index=0 ("Index")) -> (deleted portion=w686:string)  [unwired: 1 in, 1 out]
        n186 = case shown="\"f\"" w686 {
          tunnel: [w688 w689 w690] -> w675
          frame "a", Default {
            w688 = u16 0 items=["Auto", "Limited", "Fixed"] ("Gate Range\nmode 2")
          }
          frame "f" {
            w689 = u16 2 items=["Auto", "Limited", "Fixed"] ("Gate Range\nmode 2")
          }
          frame "l" {
            w690 = u16 1 items=["Auto", "Limited", "Fixed"] ("Gate Range\nmode 2")
          }
        }
      }
      frame "Error", Default {
      }
      frame "logfile" {
        n187 = Number To Decimal String(number=w705) -> (decimal integer string=w740:string)  [unwired: 1 in]
        n188 = Concatenate Strings(w739, "logfile" ("Substring"), w740, w703, ".txt" ("Substring")) -> (w737:string)
        n189 = String To Path(string=w737) -> (path=w710:path)
        n190 = Unbundle(w736) -> ("integration time"=w735:u32, "Short/Long integration time"=w734:dbl, "hold time (sec)"=w733:dbl, "delay time (sec)"=w732:dbl, "Step Time (0 disables)"=w731:dbl, "sweep method"=w730:u16, "Pulse period"=w729:dbl, "Base voltage"=w728:dbl, "Pulse width"=w727:dbl)
        n191 = Build Array(w735, w734, w733, w732, w731, w730, w729, w728, w727, w721, w722, w723, w724, w725, w726) -> (w714:dbl[])
        n192 = Insert Into Array(array=dbl[][] [] ("Input Array"), new element=w714) -> (w713:dbl[][])  [unwired: 2 in]
        n193 = call <vilib>:"compatOverwrite.vi"("overwrite (F)"=TRUE) -> ("overwrite?"=w708:T7)
        n194 = Open/Create/Replace File(file path (use dialog)=w710, error in=w712, operation (0:open)=w708) -> (refnum out=w718:refnum<file>, error out=w717:errorcluster)  [unwired: 3 in, 1 out]
        n195 = call "4155C Write array to file.vi"("Byte Stream File Refnum"=w718, "Header"=string[] ["Int Time", "Short/Long Itime", "Hold time", "Delay time", "Step time", "Sweep method", "Pulse period", "Base Voltage", "Pulse width", "Drain compliance", "Gate compliance", "Gate range mode", "Gate range", "S/D range mode", "S/D range"], "Data Array"=w713, "error in (no error)"=w717) -> ("dup refnum"=w720:refnum<file>, "error out"=w719:errorcluster)  [unwired: 1 in]
        n196 = Close File(refnum=w720, error in=w719) -> (error out=w711:errorcluster)  [unwired: 1 out]
      }
      frame "sample" {
        n197 = Number To Decimal String(number=w744) -> (decimal integer string=w792:string)  [unwired: 1 in]
        n198 = Fract/Exp String To Number(string=w789) -> (number=w750:dbl[])  [unwired: 3 in, 1 out]
        n199 = Concatenate Strings(w767, "-sample-" ("Substring"), w792, w742, ".txt" ("Substring")) -> (w790:string)
        n200 = String To Path(string=w790) -> (path=w771:path)
        n201 = Index Array(array=w750, index=0 ("Index")) -> (element=w787:dbl)
        n202 = Index Array(array=w750, index=2 ("Index")) -> (element=w783:dbl)
        n203 = Index Array(array=w750, index=3 ("Index")) -> (element=w752:dbl)
        n204 = Index Array(array=w750, index=4 ("Index")) -> (element=w749:dbl)
        n205 = call "4155C Config Sampling Measurements.vi"("Sampling interval"=w749, "Sample time"=w752, "Display on/off"=TRUE, "Timings"=w758, "Num Points"=w783, "error in (no error)"=w794, "Drain Compliance"=w793, "Gate Compliance"=w768, "VISA session"=w795) -> ("error out"=w796:errorcluster, "dup VISA resource name"=w797:refnum<visa-resource-name>)  [unwired: 1 in]
        n206 = Index Array(array=w750, index=1 ("Index")) -> (element=w784:dbl)
        n207 = call "4155C Take Sample.vi"("Emergency Stop"=w764, "error in (no error)"=w796, "Vd"=w784, "Vg"=w787, "VISA resource name in"=w797) -> ("error out"=w762:errorcluster, "Id"=w799:dbl[], "Ig"=w773:dbl[], "VISA Resource Name out"=w760:refnum<visa-resource-name>, "Is"=w798:dbl[], "Time"=w777:dbl[])  [unwired: 1 in]
        n208 = Insert Into Array(array=dbl[][] [] ("Input Array"), new element=w777) -> (w776:dbl[][])  [unwired: 2 in]
        n209 = Insert Into Array(array=w776, new element=w773) -> (w775:dbl[][])  [unwired: 2 in]
        n210 = Insert Into Array(array=w775, new element=w799) -> (w774:dbl[][])  [unwired: 2 in]
        n211 = VISA Write(VISA resource name=w760, write buffer=":DISP ON" ("write buffer (\"\")"), error in (no error)=w762) -> (VISA resource name out=w759:refnum<visa-resource-name>, error out=w761:errorcluster)  [unwired: 1 out]
        n212 = Insert Into Array(array=w774, new element=w798) -> (w766:dbl[][])  [unwired: 2 in]
        n213 = Transpose 2D Array(2D array=w766) -> (transposed array=w765:dbl[][])
        n214 = call <vilib>:"compatOverwrite.vi"("overwrite (F)"=TRUE) -> ("overwrite?"=w747:T7)
        n215 = Open/Create/Replace File(file path (use dialog)=w771, error in=w761, operation (0:open)=w747) -> (refnum out=w780:refnum<file>, error out=w779:errorcluster)  [unwired: 3 in, 1 out]
        n216 = call "4155C Write array to file.vi"("Byte Stream File Refnum"=w780, "Header"=string[] ["Time /s", "Ig /A", "Id /A", "Is /A"], "Data Array"=w765, "error in (no error)"=w779) -> ("dup refnum"=w782:refnum<file>, "error out"=w781:errorcluster)  [unwired: 1 in]
        n217 = Close File(refnum=w782, error in=w781) -> (error out=w769:errorcluster)  [unwired: 1 out]
      }
      frame "samplei" {
        n218 = Number To Decimal String(number=w801) -> (decimal integer string=w853:string)  [unwired: 1 in]
        n219 = Fract/Exp String To Number(string=w850) -> (number=w817:dbl[])  [unwired: 3 in, 1 out]
        n220 = Concatenate Strings(w832, "-samplei-" ("Substring"), w853, w800, ".txt" ("Substring")) -> (w851:string)
        n221 = String To Path(string=w851) -> (path=w835:path)
        n222 = Index Array(array=w817, index=4 ("Index")) -> (element=w811:dbl)
        n223 = Index Array(array=w817, index=3 ("Index")) -> (element=w812:dbl)
        n224 = Index Array(array=w817, index=1 ("Index")) -> (element=w814:dbl)
        n225 = Index Array(array=w817, index=0 ("Index")) -> (element=w815:dbl)
        n226 = Index Array(array=w817, index=2 ("Index")) -> (element=w813:dbl)
        n227 = call "4155C Config SamplingI Measurements.vi"("Sample time"=w813, "Display on/off"=TRUE, "Timings"=w824, "Num Points"=w814, "error in (no error)"=w855, "Sampling interval"=w812, "VISA session"=w856) -> ("error out"=w857:errorcluster, "dup VISA resource name"=w858:refnum<visa-resource-name>)  [unwired: 3 in]
        n228 = call "4155C Take SampleI.vi"("Emergency Stop"=w829, "error in (no error)"=w857, "Idg 2"=w815, "Vdg compliance 2"=w811, "VISA resource name in"=w858) -> ("error out"=w827:errorcluster, "Idg"=w860:dbl[], "Vdg"=w837:dbl[], "VISA Resource Name out"=w825:refnum<visa-resource-name>, "Is"=w859:dbl[], "Time"=w841:dbl[])  [unwired: 1 in]
        n229 = Insert Into Array(array=dbl[][] [] ("Input Array"), new element=w841) -> (w840:dbl[][])  [unwired: 2 in]
        n230 = Insert Into Array(array=w840, new element=w837) -> (w839:dbl[][])  [unwired: 2 in]
        n231 = Insert Into Array(array=w839, new element=w860) -> (w838:dbl[][])  [unwired: 2 in]
        n232 = VISA Write(VISA resource name=w825, write buffer=":DISP ON" ("write buffer (\"\")"), error in (no error)=w827) -> (VISA resource name out=w810:refnum<visa-resource-name>, error out=w826:errorcluster)  [unwired: 1 out]
        n233 = Insert Into Array(array=w838, new element=w859) -> (w831:dbl[][])  [unwired: 2 in]
        n234 = Transpose 2D Array(2D array=w831) -> (transposed array=w830:dbl[][])
        n235 = call <vilib>:"compatOverwrite.vi"("overwrite (F)"=TRUE) -> ("overwrite?"=w805:T7)
        n236 = Open/Create/Replace File(file path (use dialog)=w835, error in=w826, operation (0:open)=w805) -> (refnum out=w844:refnum<file>, error out=w843:errorcluster)  [unwired: 3 in, 1 out]
        n237 = call "4155C Write array to file.vi"("Byte Stream File Refnum"=w844, "Header"=string[] ["Time /s", "Vdg /V", "Idg /A", "Is /A"], "Data Array"=w830, "error in (no error)"=w843) -> ("dup refnum"=w846:refnum<file>, "error out"=w845:errorcluster)  [unwired: 1 in]
        n238 = Close File(refnum=w846, error in=w845) -> (error out=w808:errorcluster)  [unwired: 1 out]
        n239 = VISA Write(VISA resource name=w810, write buffer=";:PAGE:SCON:STAN OFF;:PAGE:CHAN:VSU2:DIS;" ("write buffer (\"\")"), error in (no error)=w808) -> (VISA resource name out=w806:refnum<visa-resource-name>, error out=w807:errorcluster)  [unwired: 1 out]
      }
      frame "#" {
        n240 = VISA Write(VISA resource name=w867, write buffer=":DISP ON" ("write buffer (\"\")"), error in (no error)=w866) -> (VISA resource name out=w865:refnum<visa-resource-name>, error out=w864:errorcluster)  [unwired: 1 out]
      }
      frame "stressV" {
        n241 = Number To Decimal String(number=w877) -> (decimal integer string=w918:string)  [unwired: 1 in]
        n242 = Fract/Exp String To Number(string=w915) -> (number=w888:dbl[])  [unwired: 3 in, 1 out]
        n243 = Concatenate Strings(w902, "-stressV-" ("Substring"), w918, w876, ".txt" ("Substring")) -> (w916:string)
        n244 = String To Path(string=w916) -> (path=w906:path)
        n245 = Index Array(array=w888, index=3 ("Index")) -> (element=w885:dbl)
        n246 = Index Array(array=w888, index=1 ("Index")) -> (element=w883:dbl)
        n247 = Index Array(array=w888, index=0 ("Index")) -> (element=w882:dbl)
        n248 = Index Array(array=w888, index=4 ("Index")) -> (element=w887:dbl)
        n249 = Index Array(array=w888, index=2 ("Index")) -> (element=w884:dbl)
        n250 = call "4155C Config V Stress.vi"("VISA session"=w921, "ID compliance"=w885, "VD"=w883, "VG"=w882, "IG compliance"=w884, "error in (no error)"=w920, "Display on/off"=TRUE) -> ("dup VISA resource name"=w923:refnum<visa-resource-name>, "error out"=w922:errorcluster)
        n251 = call "4155C Apply Stress.vi"("error in (no error)"=w922, "Duration"=w887, "Emergency Stop"=w901, "VISA resource name in"=w923) -> ("error out"=w899:errorcluster, "VISA Resource Name out"=w897:refnum<visa-resource-name>)
        n252 = VISA Write(VISA resource name=w897, write buffer=":DISP ON" ("write buffer (\"\")"), error in (no error)=w899) -> (VISA resource name out=w896:refnum<visa-resource-name>, error out=w898:errorcluster)  [unwired: 1 out]
        n253 = call <vilib>:"compatOverwrite.vi"("overwrite (F)"=TRUE) -> ("overwrite?"=w881:T7)
        n254 = Open/Create/Replace File(file path (use dialog)=w906, error in=w898, operation (0:open)=w881) -> (refnum out=w909:refnum<file>, error out=w908:errorcluster)  [unwired: 3 in, 1 out]
        n255 = call "4155C Write array to file.vi"("Byte Stream File Refnum"=w909, "Header"=string[] ["V stress completed successfully", ""], "error in (no error)"=w908) -> ("dup refnum"=w911:refnum<file>, "error out"=w910:errorcluster)  [unwired: 2 in]
        n256 = Close File(refnum=w911, error in=w910) -> (error out=w904:errorcluster)  [unwired: 1 out]
      }
      frame "stressI" {
        n257 = Number To Decimal String(number=w925) -> (decimal integer string=w962:string)  [unwired: 1 in]
        n258 = Fract/Exp String To Number(string=w959) -> (number=w934:dbl[])  [unwired: 3 in, 1 out]
        n259 = Concatenate Strings(w946, "-stressI-" ("Substring"), w962, w924, ".txt" ("Substring")) -> (w960:string)
        n260 = String To Path(string=w960) -> (path=w950:path)
        n261 = Index Array(array=w934, index=1 ("Index")) -> (element=w930:dbl)
        n262 = Index Array(array=w934, index=0 ("Index")) -> (element=w931:dbl)
        n263 = call "4155C Config I Stress.vi"("VISA session"=w965, "IDG"=w931, "VDG compliance"=w930, "error in (no error)"=w964, "Display on/off"=TRUE) -> ("dup VISA resource name"=w967:refnum<visa-resource-name>, "error out"=w966:errorcluster)
        n264 = Index Array(array=w934, index=2 ("Index")) -> (element=w932:dbl)
        n265 = call "4155C Apply Stress.vi"("error in (no error)"=w966, "Duration"=w932, "Emergency Stop"=w945, "VISA resource name in"=w967) -> ("error out"=w943:errorcluster, "VISA Resource Name out"=w941:refnum<visa-resource-name>)
        n266 = VISA Write(VISA resource name=w941, write buffer=":DISP ON" ("write buffer (\"\")"), error in (no error)=w943) -> (VISA resource name out=w940:refnum<visa-resource-name>, error out=w942:errorcluster)  [unwired: 1 out]
        n267 = call <vilib>:"compatOverwrite.vi"("overwrite (F)"=TRUE) -> ("overwrite?"=w929:T7)
        n268 = Open/Create/Replace File(file path (use dialog)=w950, error in=w942, operation (0:open)=w929) -> (refnum out=w953:refnum<file>, error out=w952:errorcluster)  [unwired: 3 in, 1 out]
        n269 = call "4155C Write array to file.vi"("Byte Stream File Refnum"=w953, "Header"=string[] ["I stress completed successfully", ""], "error in (no error)"=w952) -> ("dup refnum"=w955:refnum<file>, "error out"=w954:errorcluster)  [unwired: 2 in]
        n270 = Close File(refnum=w955, error in=w954) -> (error out=w948:errorcluster)  [unwired: 1 out]
      }
      frame "vsu2pulse" {
        n271 = Number To Decimal String(number=w969) -> (decimal integer string=w1004:string)  [unwired: 1 in]
        n272 = Fract/Exp String To Number(string=w1001) -> (number=w977:dbl[])  [unwired: 3 in, 1 out]
        n273 = Concatenate Strings(w989, "-vsu2-" ("Substring"), w1004, w968, ".txt" ("Substring")) -> (w1002:string)
        n274 = String To Path(string=w1002) -> (path=w993:path)
        n275 = Index Array(array=w977, index=1 ("Index")) -> (element=w976:dbl)
        n276 = Index Array(array=w977, index=0 ("Index")) -> (element=w974:dbl)
        n277 = call "4155C Config VSU2 Stress.vi"("error in (no error)"=w1006, "VSU2"=w974, "Display on/off"=TRUE, "VISA session"=w1007) -> ("error out"=w1008:errorcluster, "dup VISA resource name"=w1009:refnum<visa-resource-name>)
        n278 = call "4155C Apply Stress.vi"("error in (no error)"=w1008, "Duration"=w976, "Emergency Stop"=w988, "VISA resource name in"=w1009) -> ("error out"=w986:errorcluster, "VISA Resource Name out"=w984:refnum<visa-resource-name>)
        n279 = VISA Write(VISA resource name=w984, write buffer=":DISP ON" ("write buffer (\"\")"), error in (no error)=w986) -> (VISA resource name out=w983:refnum<visa-resource-name>, error out=w985:errorcluster)  [unwired: 1 out]
        n280 = call <vilib>:"compatOverwrite.vi"("overwrite (F)"=TRUE) -> ("overwrite?"=w973:T7)
        n281 = Open/Create/Replace File(file path (use dialog)=w993, error in=w985, operation (0:open)=w973) -> (refnum out=w996:refnum<file>, error out=w995:errorcluster)  [unwired: 3 in, 1 out]
        n282 = call "4155C Write array to file.vi"("Byte Stream File Refnum"=w996, "Header"=string[] ["VSU2 pulse completed successfully", ""], "error in (no error)"=w995) -> ("dup refnum"=w998:refnum<file>, "error out"=w997:errorcluster)  [unwired: 2 in]
        n283 = Close File(refnum=w998, error in=w997) -> (error out=w991:errorcluster)  [unwired: 1 out]
      }
      frame "sample-fpp" {
        w1022 = string[] ["Time /s", "Id VgVd /A", "Ig VgVd /A", "Vp1 VgVd /V", "Vp2 VgVd /V"] ("Header")
        w1026 = "%d" ("format string")
        n284 = Number To Decimal String(number=w1011) -> (decimal integer string=w1074:string)  [unwired: 1 in]
        n285 = Fract/Exp String To Number(string=w1071) -> (number=w1059:dbl[])  [unwired: 3 in, 1 out]
        n286 = Concatenate Strings(w1065, "-samplefpp-" ("Substring"), w1074, w1010, ".txt" ("Substring")) -> (w1072:string)
        n287 = String To Path(string=w1072) -> (path=w1034:path)
        n288 = Index Array(array=w1059, index=0 ("Index")) -> (element=w1020:dbl)
        n289 = Index Array(array=w1059, index=1 ("Index")) -> (element=w1019:dbl)
        n290 = Index Array(array=w1059, index=2 ("Index")) -> (element=w1067:dbl)
        n291 = Index Array(array=w1059, index=3 ("Index")) -> (element=w1057:dbl)
        n292 = call "4155C Config Sampling Measurements FPP.vi"("VISA session"=w1077, "Num Points"=w1067, "Vg"=w1020, "Display on/off"=TRUE, "Gate Compliance"=w1066, "Drain Compliance"=w1075, "Standby"="Standby", "error in (no error)"=w1076, "Timings"=w1064, "Vd"=w1019, "Sample time"=w1057) -> ("dup VISA resource name"=w1036:refnum<visa-resource-name>, "error out"=w1035:errorcluster)  [unwired: 3 in]
        n293 = Number To Decimal String(number=w1020) -> (decimal integer string=w1046:string)  [unwired: 1 in]
        n294 = call "4155C Take Sample FPP.vi"("VISA resource name in"=w1036, "error in (no error)"=w1035, "Emergency Stop"=w1037) -> ("Time"=w1041:dbl[], "Vp1"=w1051:dbl[], "VISA Resource Name out"=w1017:refnum<visa-resource-name>, "Ig"=w1039:dbl[], "Id"=w1040:dbl[], "Vp2"=w1049:dbl[], "error out"=w1038:errorcluster)  [unwired: 10 in]
        n295 = Insert Into Array(array=dbl[][] [] ("Input Array"), new element=w1041) -> (w1055:dbl[][])  [unwired: 2 in]
        n296 = Number To Decimal String(number=w1019) -> (decimal integer string=w1044:string)  [unwired: 1 in]
        n297 = Insert Into Array(array=w1055, new element=w1040) -> (w1054:dbl[][])  [unwired: 2 in]
        n298 = Concatenate Strings("(Vg = " ("Substring"), w1046, "V, Vd = " ("Substring"), w1044, "V)" ("Substring")) -> (w1042:string)
        n299 = Insert Into Array(array=w1054, new element=w1039) -> (w1053:dbl[][])  [unwired: 2 in]
        n300 = Insert Into Array(array=w1053, new element=w1051) -> (w1050:dbl[][])  [unwired: 2 in]
        n301 = Insert Into Array(array=w1050, new element=w1049) -> (w1018:dbl[][])  [unwired: 2 in]
        n302 = call <vilib>:"compatOverwrite.vi"("overwrite (F)"=TRUE) -> ("overwrite?"=w1015:T7)
        n303 = Open/Create/Replace File(file path (use dialog)=w1034, error in=w1038, operation (0:open)=w1015) -> (refnum out=w1031:refnum<file>, error out=w1032:errorcluster)  [unwired: 3 in, 1 out]
        n304 = Array To Spreadsheet String(array=w1022, 3:w1026) -> (spreadsheet string=w1028:string)  [unwired: 1 in]
        n305 = Transpose 2D Array(2D array=w1018) -> (transposed array=w1048:dbl[][])
        n306 = Search and Replace String(replace all?=TRUE ("replace all? (F)"), input string=w1028, search string="VgVd", replace string=w1042) -> (result string=w1024:string)  [unwired: 4 in, 3 out]
        n307 = Spreadsheet String To Array(format string=w1026, spreadsheet string=w1024, array type (2D Dbl)=w1022) -> (array=w1023:string[])  [unwired: 1 in]
        n308 = call "4155C Write array to file.vi"("Byte Stream File Refnum"=w1031, "Header"=w1023, "Data Array"=w1048, "error in (no error)"=w1032) -> ("dup refnum"=w1029:refnum<file>, "error out"=w1030:errorcluster)  [unwired: 1 in]
        n309 = Close File(refnum=w1029, error in=w1030) -> (error out=w1016:errorcluster)  [unwired: 1 out]
      }
      frame "resample-fpp" {
        w1092 = string[] ["Time /s", "Id VgVd /A", "Ig VgVd /A", "Vp1 VgVd /V", "Vp2 VgVd /V"] ("Header")
        w1096 = "%d" ("format string")
        n310 = Number To Decimal String(number=w1078) -> (decimal integer string=w1136:string)  [unwired: 1 in]
        n311 = Fract/Exp String To Number(string=w1133) -> (number=w1085:dbl[])  [unwired: 3 in, 1 out]
        n312 = Concatenate Strings(w1129, "-resamplefpp-" ("Substring"), w1136, w1079, ".txt" ("Substring")) -> (w1134:string)
        n313 = String To Path(string=w1134) -> (path=w1104:path)
        n314 = Index Array(array=w1085, index=0 ("Index")) -> (element=w1091:dbl)
        n315 = Index Array(array=w1085, index=1 ("Index")) -> (element=w1090:dbl)
        n316 = Number To Decimal String(number=w1091) -> (decimal integer string=w1114:string)  [unwired: 1 in]
        n317 = call "4155C Take Sample FPP.vi"("VISA resource name in"=w1087, "error in (no error)"=w1086, "Emergency Stop"=w1105) -> ("Time"=w1109:dbl[], "Vp1"=w1119:dbl[], "VISA Resource Name out"=w1089:refnum<visa-resource-name>, "Ig"=w1107:dbl[], "Id"=w1108:dbl[], "Vp2"=w1117:dbl[], "error out"=w1106:errorcluster)  [unwired: 10 in]
        n318 = Insert Into Array(array=dbl[][] [] ("Input Array"), new element=w1109) -> (w1123:dbl[][])  [unwired: 2 in]
        n319 = Number To Decimal String(number=w1090) -> (decimal integer string=w1112:string)  [unwired: 1 in]
        n320 = Insert Into Array(array=w1123, new element=w1108) -> (w1122:dbl[][])  [unwired: 2 in]
        n321 = Concatenate Strings("(Vg = " ("Substring"), w1114, "V, Vd = " ("Substring"), w1112, "V)" ("Substring")) -> (w1110:string)
        n322 = Insert Into Array(array=w1122, new element=w1107) -> (w1121:dbl[][])  [unwired: 2 in]
        n323 = Insert Into Array(array=w1121, new element=w1119) -> (w1118:dbl[][])  [unwired: 2 in]
        n324 = Insert Into Array(array=w1118, new element=w1117) -> (w1084:dbl[][])  [unwired: 2 in]
        n325 = call <vilib>:"compatOverwrite.vi"("overwrite (F)"=TRUE) -> ("overwrite?"=w1083:T7)
        n326 = Open/Create/Replace File(file path (use dialog)=w1104, error in=w1106, operation (0:open)=w1083) -> (refnum out=w1101:refnum<file>, error out=w1102:errorcluster)  [unwired: 3 in, 1 out]
        n327 = Array To Spreadsheet String(array=w1092, 3:w1096) -> (spreadsheet string=w1098:string)  [unwired: 1 in]
        n328 = Transpose 2D Array(2D array=w1084) -> (transposed array=w1116:dbl[][])
        n329 = Search and Replace String(replace all?=TRUE ("replace all? (F)"), input string=w1098, search string="VgVd", replace string=w1110) -> (result string=w1094:string)  [unwired: 4 in, 3 out]
        n330 = Spreadsheet String To Array(format string=w1096, spreadsheet string=w1094, array type (2D Dbl)=w1092) -> (array=w1093:string[])  [unwired: 1 in]
        n331 = call "4155C Write array to file.vi"("Byte Stream File Refnum"=w1101, "Header"=w1093, "Data Array"=w1116, "error in (no error)"=w1102) -> ("dup refnum"=w1099:refnum<file>, "error out"=w1100:errorcluster)  [unwired: 1 in]
        n332 = Close File(refnum=w1099, error in=w1100) -> (error out=w1088:errorcluster)  [unwired: 1 out]
      }
      frame "serial" {
        n333 = Index Array(array=w1140, index=0 ("Index")) -> (element=w1139:string)
        n334 = call "Serial write and read v0.4.vi"("Termination char\n(0xA = '\\n' = LF)\n(0xD = '\\r' = CR)"="Termination char\n(0xA = '\\n' = LF)\n(0xD = '\\r' = CR)", "Enable Termination\nChar (T)"="Enable Termination\nChar (T)", "parity"="parity", "stop bits"="stop bits", "string to write"=w1139, "flow control"="flow control", "byte count"="byte count", "Serial Settings:Serial End Mode for Reads"="Serial Settings:Serial End Mode for Reads", "Timeout (ms)"="Timeout (ms)", "error in (no error)"=w1145, "VISA resource name"="VISA resource name", "baud rate"="baud rate", "data bits"="data bits") -> ("read string"=→"Serial port output":string, "error out"=w1144:errorcluster)  [unwired: 1 in]
      }
    }
    n335 = Build Array("Time /s" ("element"), "Id max /A" ("VAR2 Name")) -> (w59:string[])
    n336 = Build Array(w54, w53) -> (w52:dbl[][])
    n337 = Transpose 2D Array(2D array=w52) -> (transposed array=w51:dbl[][])
    n338 = Concatenate Strings(w50, "-Ion-", ".txt" ("Suffix")) -> (w67:string)
    n339 = Array To Spreadsheet String(array=w59, 3:"" ("format string")) -> (spreadsheet string=w58:string)  [unwired: 1 in]
    n340 = Array To Spreadsheet String(array=w51, 3:"%e" ("format string")) -> (spreadsheet string=w57:string)  [unwired: 1 in]
    n341 = String To Path(string=w67) -> (path=w66:path)
    n342 = Build Array(w58, w57) -> (w56:string[])
    n343 = Write to Text File(file (use dialog)=w66, text=w56, error in=w46) -> (refnum out=w68:refnum<file>, error out=w55:errorcluster)  [unwired: 1 in, 1 out]
    n344 = Close File(refnum=w68, error in=w55) -> (error out=w45:errorcluster)  [unwired: 1 out]
    "Line running" <- w78
    "Total lines" <- w77
  }
  "error out" <- w1
